vi "LS Acquisition Main (RT).vi"() -> ()   [LabVIEW 2013]
uses:
  Type Defs/Controller List.ctl
  Type Defs/Controller Names.ctl
  Controls/Alarm Config.ctl
  Controls/Alarm Definition.ctl
  Controls/Alarm Profile Config.ctl
  Controls/Tank CMDs.ctl
  Controls/Controller Config.ctl
  Controls/Pump Data.ctl
  Controls/Tank Data.ctl
  Controls/HMI Cluster.ctl
  Controls/HMI Header.ctl
  Controls/HMI Tog Buttons.ctl
  Controls/HMI Mom Buttons.ctl
  Type Defs/LS Data.ctl
  Type Defs/Sequence States.ctl
  Type Defs/LS DAS App Config.ctl
  SubVIs/Data Logger/Data Log Init.ctl
  Controls/App Global Mode.ctl
  <vilib>/FPGAPlugInAG/sbRIO-9626/niLvFpga_Open_sbRIO-9626.vi
  <vilib>/Utility/error.llb/Error Cluster From Error Code.vi
  <vilib>/rvi/errors/niLvFpgaAdjustHostInterfaceError.vi
  <vilib>/rvi/interface/nirviOpenFPGA/nirviOpenFPGA.xnode
  FPGA Bitfiles/LS Acquisition.lvbitx
  <vilib>/rvi/interface/nirviReadWriteControl/nirviReadWriteControl.xnode
  <vilib>/Utility/config.llb/NI_LVConfig.lvlib
  <vilib>/rvi/errors/niLvFpgaMergeErrorWithErrorCode.vi
  NiFpgaLv.dll
panel:
  in  "Data File Name:":string caption="*Data File Name:"
  in  "pb.Run Profile":bool
  in  "Bank 2":T1={"7"=TRUE, "8"=TRUE, "9"=TRUE, "10"=TRUE, "11"=TRUE}
  in  "Bank 1":T2={"1"=TRUE, "2"=TRUE, "3"=TRUE, "4"=TRUE, "5"=TRUE} caption="Present"
  out "Recording":bool
  out "Cycles Completed:":u32=17
  out "Read Inputs (ms)":u32
  out "Update Screen (ms)":u32
  out "Run Step (ms)":u32
  in  "Reset Tab":enum32{"Page 1", "Page 2"}(tab)
  in  "pb.Reset OK":bool
  in  "pb.Reset Cancel":bool
  in  "Save As Tab":enum32{"Page 1", "Page 2"}(tab)
  in  "New Profile Name:":string
  in  "pb.Save As OK":bool
  in  "pb.Save As Cancel":bool
  in  "Alarm Tab":enum32{"Page 1", "Page 2"}(tab)
  in  "Set Time Tab":enum32{"Page 1", "Page 2"}(tab)
  in  "Pump Timers Tab":enum32{"Page 2"}(tab)
  in  "LS Serial Numbers":T3 caption="Serial Numbers"
  out "CPU Usage:":dbl=7.74131899555212 format="%.1f"
  in  "Live Data Tab":enum32{"Page 2", "Page 3"}(tab)=enum."Page 3"
  in  "Reset Anomalies":bool
  in  "Reset Total Cycles":bool
  out "Anomalies (Last Cycle)":i32[](array[numeric]) caption="Anomalies\n(Last Cycle)" format="%#.0f"
  out "Anomalies/Cycle":i32[](array[numeric]) caption="Anomalies/\nCycle" format="%#.0f"
  out "Cycles":u32[](array[numeric]) caption="Powered\nCycles" format="%#.0f"
  out "Anomalies Total":i32[](array[numeric]) caption="Anomalies\nTotal" format="%#.0f"
  out "Steps":u32[](array[numeric]) format="%#.0f"
  out "Total Cycles":u32[](array[numeric]) caption="Total\nPowered\nCycles" format="%#.0f"
  out "Replace SD Card":bool=TRUE
  out "SD Card % Usage":dbl format="%.2g"
  in  "Reset Opens":bool
  out "Opens":i32[](array[numeric]) format="%#.0f"
  in  "Title Tab":enum32{"Page 1", "Page 2"}(tab)
  in  "Title":string="LS Data Acquisition System, v1.9"
  out "Time/Date":string
  in  "Login":bool
  in  "pb.Stop Profile":bool
  in  "Main Tab":enum32{"Main", "Live Graph", "Configure"}(tab)
  in  "Profile based record":bool
  in  "Detection Mode:":u16(ring) items=["Vibration", "Slosh", "Dirt"]
  in  "LS Cycle Time (ms):":dbl=244.0 min=0.1 max=1000.0 step=0.1
  in  "LS On Time (ms):":dbl=4.0 min=0.0 max=1000.0 step=0.01
  in  "Bank 2 Power State:":u16(ring) items=["0 - Off", "1 - On", "2 - Pulsing"]
  in  "Bank 1 Power State:":u16(ring) items=["0 - Off", "1 - On", "2 - Pulsing"]
  in  "CA Number:":string
  in  "Profile Name:":string(combo)="test"
  in  "pb.Save As":bool
  out "Location:":string
  in  "Profile:":string[][](table)=[["1", "216000", "1", "2", "244", "4", "1", "67.6"], ["2", "1800", "0", "0", "244", "4", "1", "10.0"], ["3", "39600", "0", "0", "244", "4", "0", ""], ["4", "1800", "0", "0", "244", "4", "1", ""]]
  out "Recording":bool
  out "Step:":i32=2
  out "Time Left:":dbl=0.21101045608520508
  in  "Bank 2 Record Rate (hz)":enum16{"4.37", "1000"}(ring)
  in  "Graph Selection":T4(ring)
  out "Waveform Chart":dbl(graph)
  in  "Pause":bool
  in  "Bank 2 Voltage Offset:":dbl min=0.0 max=999999.0 step=1.0
  in  "Bank 1 Voltage Offset:":dbl min=0.0 max=999999.0 step=1.0
  in  "Cycle Pts to Avg:":i32=20 min=0 max=999999 step=1
  in  "Cycle Threshold:":dbl=1.6 min=0.0 max=999999.0 step=1.0
  in  "Note Tab":enum32{"Page 1", "Page 2"}(tab)
  in  "Stop Profile Note":string
  in  "pb.Note OK":bool
  in  "pb.Note Cancel":bool
  # "Are you sure you want to reset?"
  # "Enter a new elapsed time."
  # "Level Sensor Monitor"
  # "Level Sensor Monitor"
  # "Have not finished debug:\n     check open log\n     should a profile time stop be added\n     watch CPU, nearing limit"
  # "Record Rate=1kHz"
  # "*"
  # "*"
  # "Data file note as to reason for stopping profile:"
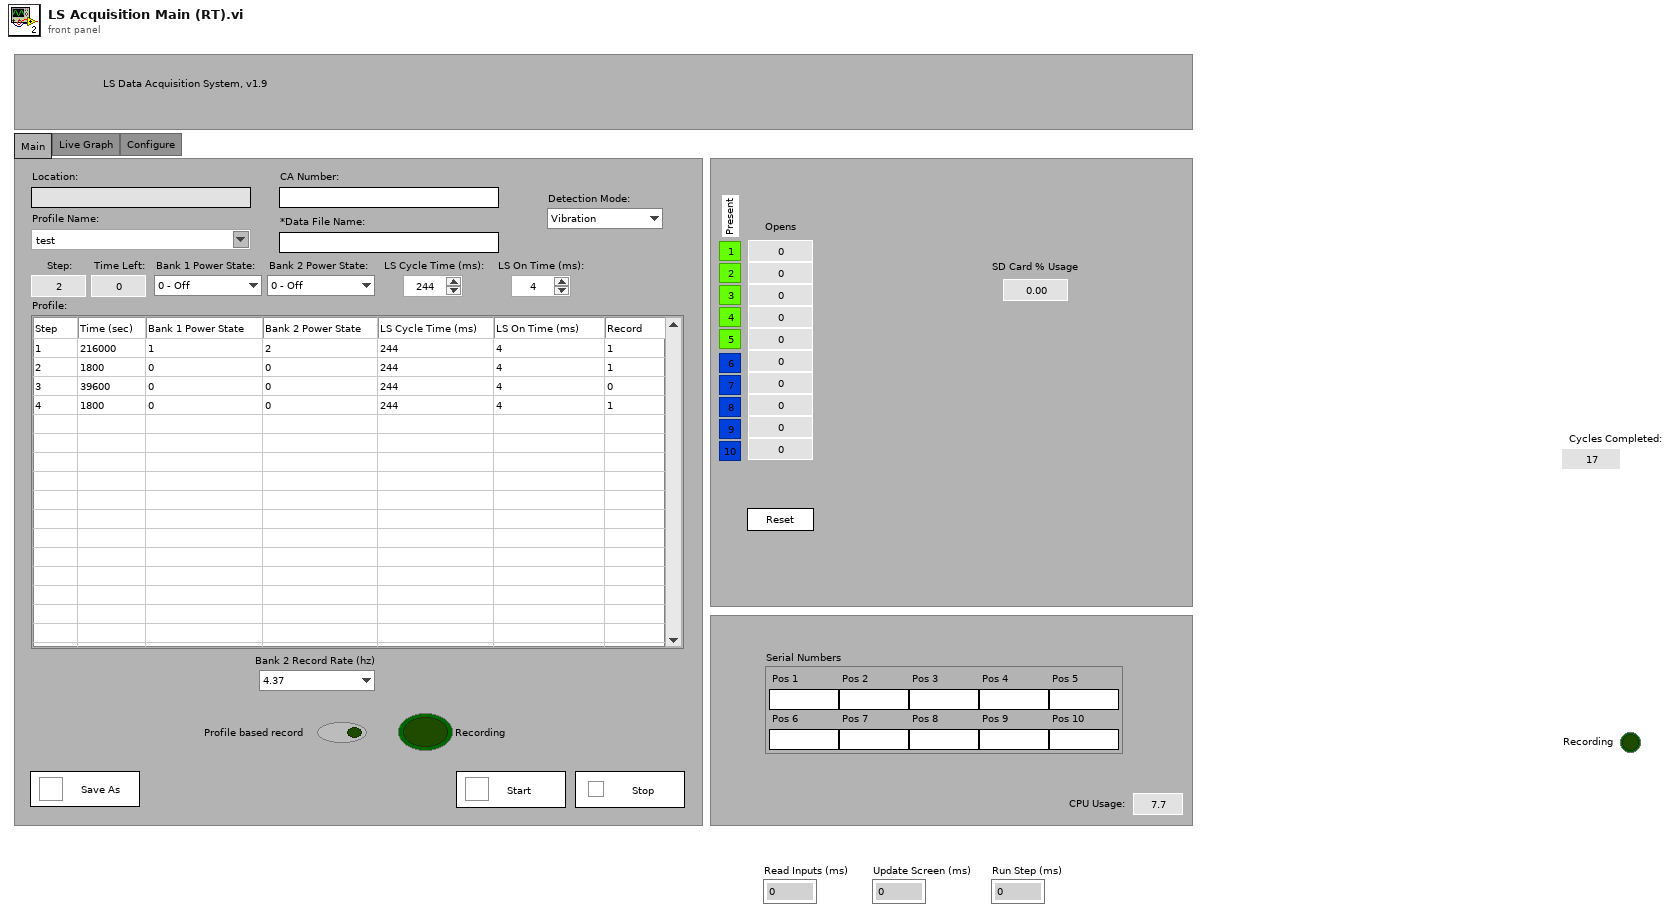
[diagram p1: front panel]
types:
  T1 = cluster{"7":bool, "8":bool, "9":bool, "10":bool, "11":bool}
  T2 = cluster{"1":bool, "2":bool, "3":bool, "4":bool, "5":bool}
  T3 = cluster{"Pos 1":string, "Pos 2":string, "Pos 3":string, "Pos 4":string, "Pos 5":string, "Pos 6":string, "Pos 7":string, "Pos 8":string, "Pos 9":string, "Pos 10":string}
  T4 = enum16{"Pos 1", "Pos 2", "Pos 3", "Pos 4", "Pos 5", "Pos 6", "Pos 7", "Pos 8", "Pos 9", "Pos 10", "Power Supply"}
  T5 = typedef "LS DAS App Config.ctl" = cluster{"Location":string, "Profiles Path":path, "Current Profile":string, "CA Number":string, "Cycles Completed":u32, "Stagger Time (ms)":i32, "Pumps Present":cluster{"Pump 1":bool, "Pump 2":bool, "Pump 3":bool, "Pump 4":bool, "Pump 5":bool, "Pump 6":bool}, "Data Log Init":T6, "Email Handler IP":string, "Cycle Threshold:":dbl, "Cycle Pts to Avg:":i32, "Anomaly Threshold:":dbl, "Normal Steps:":u32, "Step Threshold:":dbl, "Bank 1 Offset":dbl, "Bank 2 Offset":dbl, "LS Power (Freq):":dbl, "LS Power (Duty):":dbl, "Bank 1 Present":cluster{"1":bool, "2":bool, "3":bool, "4":bool, "5":bool}, "Bank 2 Present":cluster{"6":bool, "7":bool, "8":bool, "9":bool, "10":bool}, "Data File Name":string, "Detection Mode":i32, "Serial Numbers":string[], "Profile Record":bool, "Bank2 Record Rate":u16}
  T6 = typedef "Data Log Init.ctl" = cluster{"Data Path":path, "Data Log Rate (S/s)":u32, "AKLH Rate (Hours/S)":dbl, "Sync Time Offset (min)":i32, "IP Last 3":i32, "WebDAV IP":string}
  T7 = typedef "Sequence States.ctl" = enum16{"Main", "Init Files", "Init", "Unused", "Save As", "Start Profile", "Check Step Time", "Alarm", "Alarm Dismiss", "Run Step", "Stop Profile", "Cycle Reset", "Time Reset", "Time Reset All", "Time Set", "Tare CTs", "Save Profile", "Open Profile", "Get Profiles", "Update Screen", "Update Controls", "Save App Config", "Write Outputs", "Disable Background", "Enable Background", "Get/Release Control", "Log Fuel Change", "Fuel Change Popup", "Read Inputs", "Remote Timer Reset", "Controller Change", "Get Alarms", "Init Alarms", "Save Alarms", "Voltage Selection", "Set Watlow Temp 1", "Set Watlow Temp 2", "Get Pressure", "Write Tare Pressure", "Adjust Controls", "Reinit ADC", "Write Initial Times", "Write Pumps Present", "HMI Command", "Save Pump Times", "Check Pump Stop Time", "Save LS App Config", "Init Data File", "Reset LS Cycles", "Reset Anomalies", "Reset Opens", "Save LS Data", "Save LS Test Data", "Check Serial Numbers", "Main Tab", "Allow Data Note", "Resume Profile", "Pause Profile", "Allow Pause Note", "Clear Graph"}
  T8 = typedef "LS Data.ctl" = cluster{"Total Cycles":u32[], "Steps":u32[], "Anomalies Total":i32[], "Cycles":u32[], "Anomalies/Cycle":i32[], "Anomalies (Last Cycle)":i32[], "Opens":i32[]}
  T9 = typedef "HMI Cluster.ctl" = cluster{"Error":errorcluster, "COM Ref":refnum<visa-resource-name>, "Pump Data":T10, "Tank Data":cluster{"PS Actual (V):":dbl, "Temp1":dbl, "Temp2":dbl}, "Power Relays":cluster{"Pump 1":bool, "Pump 2":bool, "Pump 3":bool, "Pump 4":bool, "Pump 5":bool, "Pump 6":bool}, "Pump CMDs":dbl[], "HMI Header":T11, "Tank CMDs":T12, "HMI Tog Buttons":T13, "In Test":bool, "HMI Command":bool, "HMI Mom Buttons":T14, "Controller Config":T15, "Alarm":bool, "Alarm Message 1":string, "Alarm Message 2":string, "Recording":bool, "Serial Numbers":string[], "Pumps Present":bool[]}
  T10 = typedef "Pump Data.ctl" = cluster{"Voltages":dbl[], "PumpCurrent":dbl[], "Speed":dbl[], "ControllerCurrent":dbl[], "Pressure":dbl[], "Flow":dbl[], "Elapsed Time (Display)":dbl[], "Avg Pressure":dbl, "Avg Speed":dbl, "Elapsed Time":dbl[]}
  T11 = typedef "HMI Header.ctl" = cluster{"Line 1":string, "Line 2":string, "Line 3":string, "Line 4":string}
  T12 = typedef "Tank CMDs.ctl" = cluster{"PS CMD":dbl, "Press CMD":dbl, "Temp 1 CMD":dbl, "Temp 2 CMD":dbl}
  T13 = typedef "HMI Tog Buttons.ctl" = cluster{"Start Test":bool, "Toggle Spare 1":bool, "Toggle Spare 2":bool, "Toggle Spare 3":bool, "Toggle Spare 4":bool, "Toggle Spare 5":bool}
  T14 = typedef "HMI Mom Buttons.ctl" = cluster{"Stop":bool, "Reset Timers":bool, "Log Fuel Change":bool, "Alarm Dismiss":bool}
  T15 = typedef "Controller Config.ctl" = cluster{"Controller Name":T16, "CommSeg":i32, "PWM?":bool, "Frequency":i32, "Low Command":dbl, "High Command":dbl, "Stop Command":dbl, "Command Step":dbl, "Solenoid Stop?":bool, "Controller?":bool, "Invert PWM":bool}
  T16 = typedef "Controller Names.ctl" = enum16{"Kuhnke", "Helbako BLDC", "Conti", "Hella BLDC OL PWM", "Hella BLDC Turbine OL PWM", "Hella BLDC Pressure", "Helbako (old)", "TI PWM", "PSA", "Hella Gas", "Hella Diesel", "8 Comm", "10 Comm", "8 Comm Hella", "10 Comm Hella", "8 Comm Omron", "10 Comm Omron", "8 Comm Nissan", "10 Comm Nissan"}
  T17 = typedef "Tank Data.ctl" = cluster{"PS Actual (V):":dbl, "Temp1":dbl, "Temp2":dbl}
  T18 = typedef "Alarm Config.ctl" = cluster{"Alarms:":T19[], "Profile Sync:":T20}
  T19 = typedef "Alarm Definition.ctl" = cluster{"Description:":string, "Enabled:":bool, "Data Index:":i32, "Data Type:":string, "Low Limit:":dbl, "High Limit:":dbl, "Trip Time:":u32, "Profile Sync:":bool}
  T20 = typedef "Alarm Profile Config.ctl" = cluster{"Trip Time:":u32, "Consecutive Trips:":i32}
  T21 = typedef "Controller List.ctl" = cluster{"Controller Name":T16, "CommSeg":i32, "PWM?":bool, "Frequency":i32, "Low Command":dbl, "High Command":dbl, "Stop Command":dbl, "Command Step":dbl, "Solenoid Stop?":bool, "Controller?":bool, "Invert PWM":bool}[]
  T22 = cluster{"Pump 1":bool, "Pump 2":bool, "Pump 3":bool, "Pump 4":bool, "Pump 5":bool, "Pump 6":bool}
  T23 = cluster{"Error":errorcluster, "Profile":string[][], "LS DAS Config":T5, "Profiles":string[], "Current Step":i32, "Step Time Left":dbl, "Run Profile":bool, "Step Start Time":dbl, "Step Time":dbl, " # of Steps":i32, "Screen Timer":u32, "Last Profile Time":dbl, "Controller CMDs":dbl[], "Client?":bool, "pb.Run Profile":bool, "pb.Resets":bool[], "pb.Sets":bool[], "Initial Times":dbl[], "Pressure Offsets":dbl[], "Login":bool, "Stagger Counter":i32, "New Step":bool, "Inputs Timer":u32, "Tank Data":T17, "Voltage Enable":bool, "Power Relay":cluster{"Pump 1":bool, "Pump 2":bool, "Pump 3":bool, "Pump 4":bool, "Pump 5":bool, "Pump 6":bool}, "Ignition Relay":cluster{"Pump 1":bool, "Pump 2":bool, "Pump 3":bool, "Pump 4":bool, "Pump 5":bool, "Pump 6":bool}, "Controller List":T21, "Alarm Config":T18, "Alarm Config Path":path, "Trip Counters":i32[], "Previous Times":u32[], "Alarm Message 1":string, "Alarm Message 2":string, "Prev ON Times":u32[], "CalArray":dbl[][], "Tank CMDs":T12, "Controller Config":T15, "Fuel Log Path":path, "Pump Data":T10, "Alarm Latch":bool, "Time/Date":string, "Recording":bool, "HMI":T9, "WebDAV Push":bool, "Email Alarms Disabled":bool, "Concat Data":bool, "LS Data":T8, "Main Tab":enum32{"Main", "Live Graph", "Configure"}, "Bank 1 State:":u16, "Bank 2 State:":u16, "LS Data Filepath":path, "Initial LS Data":T8, "day of month":i32, "Pause Test":bool, "ProfileMinute":i32, "Record Step":bool, "Graph Selection":enum16{"Pos 1", "Pos 2", "Pos 3", "Pos 4", "Pos 5", "Pos 6", "Pos 7", "Pos 8", "Pos 9", "Pos 10", "Power Supply"}, "Graph Pause":bool}
  T24 = typedef "App Global Mode.ctl" = enum16{"Read", "Write Client", "Write Login"}
  T25 = enum16{"Read", "Engine Writes", "Main Writes", "Write Anomalies", "Write Init Data", "Write Storage", "Write Note", "Read Note"}
  T26 = cluster{"Running?":bool, "Record":bool, "Data Filepath":path, "Serial Numbers":string[]}
  T27 = enum32{"Main", "Live Graph", "Configure", "Alarms", "Advanced"}
  T28 = enum8{"Enabled", "Disabled", "Disabled and Grayed Out"}
  T29 = cluster{"6":bool, "7":bool, "8":bool, "9":bool, "10":bool}
  T30 = typedef "NI_LVConfig.lvlib/Config Data RefNum.ctl" = refnum<k1>
  T31 = typedef "LVDateTimeRec.ctl" = cluster{"fractional second":dbl, "second":i32, "minute":i32, "hour":i32, "day of month":i32, "month":i32, "year":i32, "day of week":i32, "day of year":i32, "DST":i32}
  T32 = cluster{"Serial Numbers[0]":string, "Serial Numbers[1]":string, "Serial Numbers[2]":string, "Serial Numbers[3]":string, "Serial Numbers[4]":string, "Serial Numbers[5]":string, "Serial Numbers[6]":string, "Serial Numbers[7]":string, "Serial Numbers[8]":string, "Serial Numbers[9]":string}
  T33 = cluster{"[0]":string, "[1]":string, "[2]":string, "[3]":string, "[4]":string, "[5]":string, "[6]":string, "[7]":string, "[8]":string, "[9]":string}
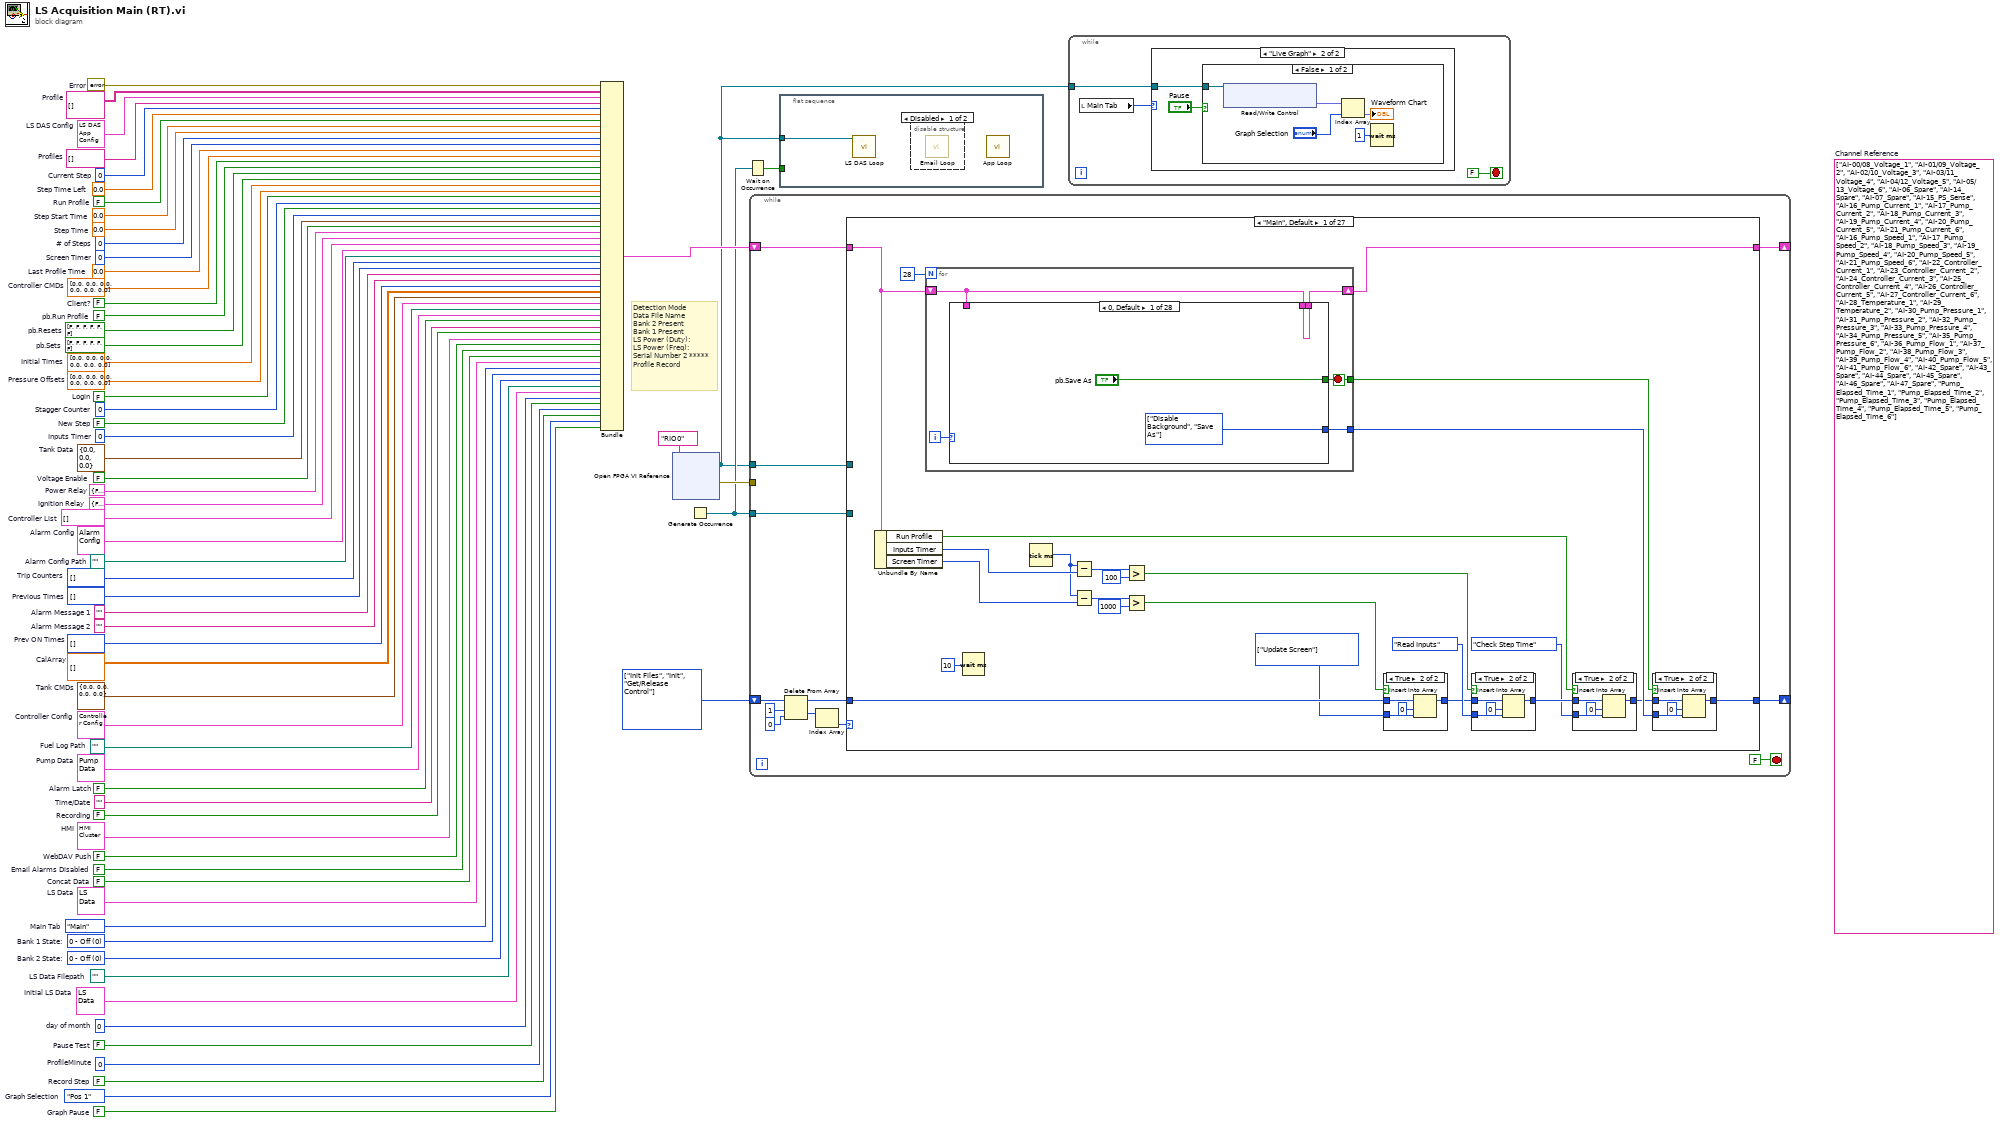
[diagram p0: block diagram]
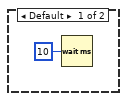
[diagram p2: hidden frame]
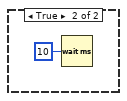
[diagram p3: hidden frame]
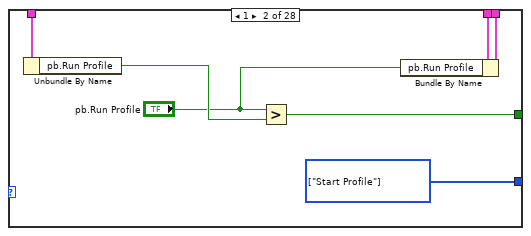
[diagram p9: hidden frame]
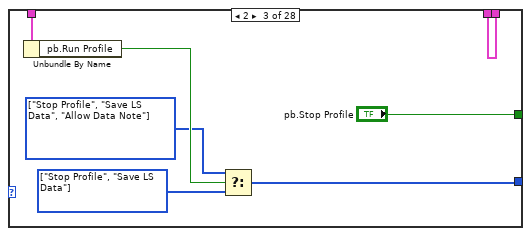
[diagram p10: hidden frame]
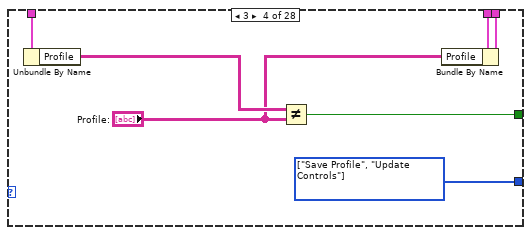
[diagram p11: hidden frame]
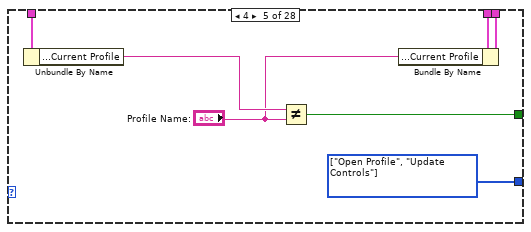
[diagram p12: hidden frame]
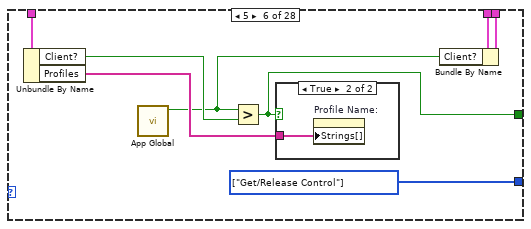
[diagram p13: hidden frame]
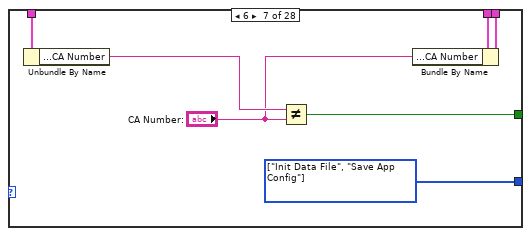
[diagram p15: hidden frame]
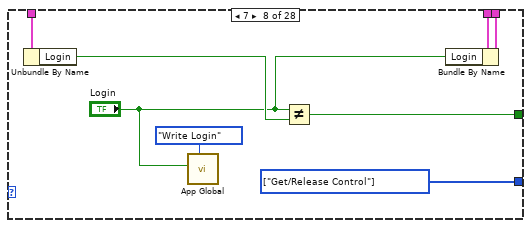
[diagram p16: hidden frame]
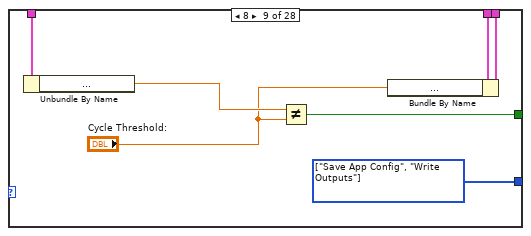
[diagram p17: hidden frame]
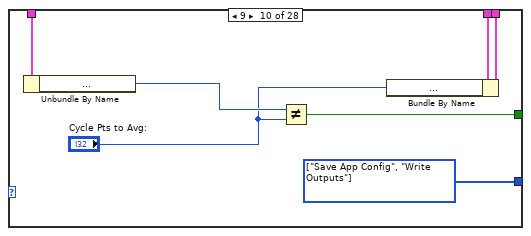
[diagram p18: hidden frame]
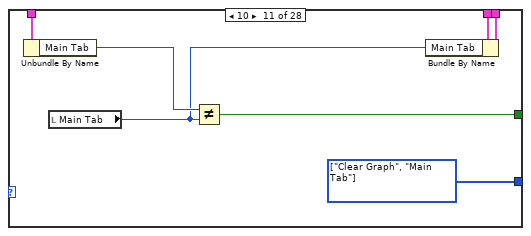
[diagram p19: hidden frame]
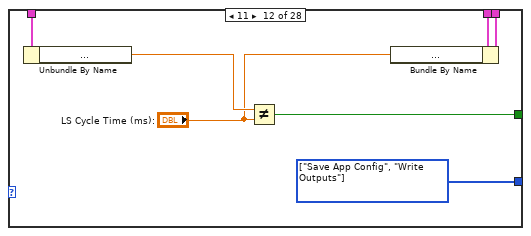
[diagram p20: hidden frame]
diagram:
  w1 = FALSE  # Graph Pause
  w2 = T4."Pos 1"  # Graph Selection
  w3 = enum32{"Main", "Live Graph", "Configure"}."Main"  # Main Tab
  w4 = FALSE  # Record Step
  w5 = T5 {"Location"="", "Profiles Path"=path "", "Current Profile"="", "CA Number"="", "Cycles Completed"=0, "Stagger Time (ms)"=0, "Pumps Present"={"Pump 1"=FALSE, "Pump 2"=FALSE, "Pump 3"=FALSE, "Pump 4"=FALSE, "Pump 5"=FALSE, "Pump 6"=FALSE}, "Data Log Init"={"Data Path"=path "", "Data Log Rate (S/s)"=0, "AKLH Rate (Hours/S)"=0.0, "Sync Time Offset (min)"=0, "IP Last 3"=0, "WebDAV IP"=""}, "Email Handler IP"="", "Cycle Threshold:"=0.0, "Cycle Pts to Avg:"=0, "Anomaly Threshold:"=0.0, "Normal Steps:"=0, "Step Threshold:"=0.0, "Bank 1 Offset"=0.0, "Bank 2 Offset"=0.0, "LS Power (Freq):"=0.0, "LS Power (Duty):"=0.0, "Bank 1 Present"={"1"=FALSE, "2"=FALSE, "3"=FALSE, "4"=FALSE, "5"=FALSE}, "Bank 2 Present"={"6"=FALSE, "7"=FALSE, "8"=FALSE, "9"=FALSE, "10"=FALSE}, "Data File Name"="", "Detection Mode"=0, "Serial Numbers"=[], "Profile Record"=FALSE, "Bank2 Record Rate"=0}  # LS DAS Config
  w6 = 0  # ProfileMinute
  w7 = FALSE  # Pause Test
  w8 = 0  # day of month
  (unwired) string[] ["AI-00/08_Voltage_1", "AI-01/09_Voltage_2", "AI-02/10_Voltage_3", "AI-03/11_Voltage_4", "AI-04/12_Voltage_5", "AI-05/13_Voltage_6", "AI-06_Spare", "AI-14_Spare", "AI-07_Spare", "AI-15_PS_Sense", "AI-16_Pump_Current_1", "AI-17_Pump_Current_2", "AI-18_Pump_Current_3", "AI-19_Pump_Current_4", "AI-20_Pump_Current_5", "AI-21_Pump_Current_6", "AI-16_Pump_Speed_1", "AI-17_Pump_Speed_2", "AI-18_Pump_Speed_3", "AI-19_Pump_Speed_4", "AI-20_Pump_Speed_5", "AI-21_Pump_Speed_6", "AI-22_Controller_Current_1", "AI-23_Controller_Current_2", "AI-24_Controller_Current_3", "AI-25_Controller_Current_4", "AI-26_Controller_Current_5", "AI-27_Controller_Current_6", "AI-28_Temperature_1", "AI-29_Temperature_2", "AI-30_Pump_Pressure_1", "AI-31_Pump_Pressure_2", "AI-32_Pump_Pressure_3", "AI-33_Pump_Pressure_4", "AI-34_Pump_Pressure_5", "AI-35_Pump_Pressure_6", "AI-36_Pump_Flow_1", "AI-37_Pump_Flow_2", "AI-38_Pump_Flow_3", "AI-39_Pump_Flow_4", "AI-40_Pump_Flow_5", "AI-41_Pump_Flow_6", "AI-42_Spare", "AI-43_Spare", "AI-44_Spare", "AI-45_Spare", "AI-46_Spare", "AI-47_Spare", "Pump_Elapsed_Time_1", "Pump_Elapsed_Time_2", "Pump_Elapsed_Time_3", "Pump_Elapsed_Time_4", "Pump_Elapsed_Time_5", "Pump_Elapsed_Time_6"]  # Channel Reference
  w14 = T7[] [enum."Init Files", enum."Init", enum."Get/Release Control"] items=["Main", "Init Files", "Init", "Unused", "Save As", "Start Profile", "Check Step Time", "Alarm", "Alarm Dismiss", "Run Step", "Stop Profile", "Cycle Reset", "Time Reset", "Time Reset All", "Time Set", "Tare CTs", "Save Profile", "Open Profile", "Get Profiles", "Update Screen", "Update Controls", "Save App Config", "Write Outputs", "Disable Background", "Enable Background", "Get/Release Control", "Log Fuel Change", "Fuel Change Popup", "Read Inputs", "Remote Timer Reset", "Controller Change", "Get Alarms", "Init Alarms", "Save Alarms", "Voltage Selection", "Set Watlow Temp 1", "Set Watlow Temp 2", "Get Pressure", "Write Tare Pressure", "Adjust Controls", "Reinit ADC", "Write Initial Times", "Write Pumps Present", "HMI Command", "Save Pump Times", "Check Pump Stop Time", "Save LS App Config", "Init Data File", "Reset LS Cycles", "Reset Anomalies", "Reset Opens", "Save LS Data", "Save LS Test Data", "Check Serial Numbers", "Main Tab", "Allow Data Note", "Resume Profile", "Pause Profile", "Allow Pause Note", "Clear Graph"]
  w15 = T8 {"Total Cycles"=[0, 0, 0, 0, 0, 0, 0, 0, 0, 0, 0, 0], "Steps"=[0, 0, 0, 0, 0, 0, 0, 0, 0, 0, 0, 0], "Anomalies Total"=[0, 0, 0, 0, 0, 0, 0, 0, 0, 0, 0, 0], "Cycles"=[0, 0, 0, 0, 0, 0, 0, 0, 0, 0, 0, 0], "Anomalies/Cycle"=[0, 0, 0, 0, 0, 0, 0, 0, 0, 0, 0, 0], "Anomalies (Last Cycle)"=[0, 0, 0, 0, 0, 0, 0, 0, 0, 0, 0, 0], "Opens"=[0, 0, 0, 0, 0, 0, 0, 0, 0, 0, 0, 0]}  # Initial LS Data
  w16 = path ""  # LS Data Filepath
  w18 = u16 0 items=["0 - Off", "1 - On", "2 - Pulsing"]  # Bank 1 State:
  w17 = u16 0 items=["0 - Off", "1 - On", "2 - Pulsing"]  # Bank 2 State:
  w19 = T8 {"Total Cycles"=[0, 0, 0, 0, 0, 0, 0, 0, 0, 0, 0, 0], "Steps"=[0, 0, 0, 0, 0, 0, 0, 0, 0, 0, 0, 0], "Anomalies Total"=[0, 0, 0, 0, 0, 0, 0, 0, 0, 0, 0, 0], "Cycles"=[0, 0, 0, 0, 0, 0, 0, 0, 0, 0, 0, 0], "Anomalies/Cycle"=[0, 0, 0, 0, 0, 0, 0, 0, 0, 0, 0, 0], "Anomalies (Last Cycle)"=[0, 0, 0, 0, 0, 0, 0, 0, 0, 0, 0, 0], "Opens"=[]}  # LS Data
  w20 = FALSE  # Concat Data
  w21 = FALSE  # Email Alarms Disabled
  w22 = FALSE  # WebDAV Push
  w23 = T9 {"Error"={"status"=FALSE, "code"=0, "source"=""}, "COM Ref"="", "Pump Data"={"Voltages"=[], "PumpCurrent"=[], "Speed"=[], "ControllerCurrent"=[], "Pressure"=[], "Flow"=[], "Elapsed Time (Display)"=[], "Avg Pressure"=0.0, "Avg Speed"=0.0, "Elapsed Time"=[]}, "Tank Data"={"PS Actual (V):"=0.0, "Temp1"=0.0, "Temp2"=0.0}, "Power Relays"={"Pump 1"=FALSE, "Pump 2"=FALSE, "Pump 3"=FALSE, "Pump 4"=FALSE, "Pump 5"=FALSE, "Pump 6"=FALSE}, "Pump CMDs"=[], "HMI Header"={"Line 1"="", "Line 2"="", "Line 3"="", "Line 4"=""}, "Tank CMDs"={"PS CMD"=0.0, "Press CMD"=0.0, "Temp 1 CMD"=0.0, "Temp 2 CMD"=0.0}, "HMI Tog Buttons"={"Start Test"=FALSE, "Toggle Spare 1"=FALSE, "Toggle Spare 2"=FALSE, "Toggle Spare 3"=FALSE, "Toggle Spare 4"=FALSE, "Toggle Spare 5"=FALSE}, "In Test"=FALSE, "HMI Command"=FALSE, "HMI Mom Buttons"={"Stop"=FALSE, "Reset Timers"=FALSE, "Log Fuel Change"=FALSE, "Alarm Dismiss"=FALSE}, "Controller Config"={"Controller Name"=enum."Kuhnke", "CommSeg"=0, "PWM?"=FALSE, "Frequency"=0, "Low Command"=0.0, "High Command"=0.0, "Stop Command"=0.0, "Command Step"=0.0, "Solenoid Stop?"=FALSE, "Controller?"=FALSE, "Invert PWM"=FALSE}, "Alarm"=FALSE, "Alarm Message 1"="", "Alarm Message 2"="", "Recording"=FALSE, "Serial Numbers"=[], "Pumps Present"=[]}  # HMI
  w24 = T17 {"PS Actual (V):"=0.0, "Temp1"=0.0, "Temp2"=0.0}  # Tank Data
  w25 = FALSE  # Recording
  w26 = ""  # Time/Date
  w27 = ""  # Alarm Message 2
  w28 = FALSE  # Alarm Latch
  w29 = T10 {"Voltages"=[0.015201568603515625, 0.00335693359375, 0.003021240234375, 0.12260055541992188, 0.06085968017578125, 0.052234649658203125], "PumpCurrent"=[0.015201568603515625, 0.00335693359375, 0.003021240234375, 0.12260055541992188, 0.06085968017578125, 0.052234649658203125], "Speed"=[0.0, 0.0, 0.0, 0.0, 0.0, 0.0], "ControllerCurrent"=[0.015201568603515625, 0.00335693359375, 0.003021240234375, 0.12260055541992188, 0.06085968017578125, 0.052234649658203125], "Pressure"=[0.015201568603515625, 0.00335693359375, 0.003021240234375, 0.12260055541992188, 0.06085968017578125, 0.052234649658203125], "Flow"=[0.0, 0.0, 0.0, 0.125, 0.0625, 0.0625], "Elapsed Time (Display)"=[7.1, 7.1, 7.1, 458133.45, 458138.85000000003, 458126.75], "Avg Pressure"=0.0, "Avg Speed"=0.0, "Elapsed Time"=[]}  # Pump Data
  w30 = path ""  # Fuel Log Path
  w31 = T15 {"Controller Name"=enum."Kuhnke", "CommSeg"=0, "PWM?"=FALSE, "Frequency"=0, "Low Command"=0.0, "High Command"=0.0, "Stop Command"=0.0, "Command Step"=0.0, "Solenoid Stop?"=FALSE, "Controller?"=FALSE, "Invert PWM"=FALSE}  # Controller Config
  w32 = T12 {"PS CMD"=0.0, "Press CMD"=0.0, "Temp 1 CMD"=0.0, "Temp 2 CMD"=0.0}  # Tank CMDs
  w33 = dbl[][] []  # CalArray
  w34 = u32[] []  # Prev ON Times
  w35 = ""  # Alarm Message 1
  w36 = u32[] []  # Previous Times
  w37 = i32[] []  # Trip Counters
  w38 = path ""  # Alarm Config Path
  w39 = T18 {"Alarms:"=[{"Description:"="", "Enabled:"=FALSE, "Data Index:"=0, "Data Type:"="", "Low Limit:"=0.0, "High Limit:"=0.0, "Trip Time:"=0, "Profile Sync:"=FALSE}, {"Description:"="", "Enabled:"=FALSE, "Data Index:"=0, "Data Type:"="", "Low Limit:"=0.0, "High Limit:"=0.0, "Trip Time:"=0, "Profile Sync:"=FALSE}, {"Description:"="", "Enabled:"=FALSE, "Data Index:"=0, "Data Type:"="", "Low Limit:"=0.0, "High Limit:"=0.0, "Trip Time:"=0, "Profile Sync:"=FALSE}, {"Description:"="", "Enabled:"=FALSE, "Data Index:"=0, "Data Type:"="", "Low Limit:"=0.0, "High Limit:"=0.0, "Trip Time:"=0, "Profile Sync:"=FALSE}, {"Description:"="", "Enabled:"=FALSE, "Data Index:"=0, "Data Type:"="", "Low Limit:"=0.0, "High Limit:"=0.0, "Trip Time:"=0, "Profile Sync:"=FALSE}, {"Description:"="", "Enabled:"=FALSE, "Data Index:"=0, "Data Type:"="", "Low Limit:"=0.0, "High Limit:"=0.0, "Trip Time:"=0, "Profile Sync:"=FALSE}, {"Description:"="", "Enabled:"=FALSE, "Data Index:"=0, "Data Type:"="", "Low Limit:"=0.0, "High Limit:"=0.0, "Trip Time:"=0, "Profile Sync:"=FALSE}, {"Description:"="", "Enabled:"=FALSE, "Data Index:"=0, "Data Type:"="", "Low Limit:"=0.0, "High Limit:"=0.0, "Trip Time:"=0, "Profile Sync:"=FALSE}], "Profile Sync:"={"Trip Time:"=0, "Consecutive Trips:"=0}}  # Alarm Config
  w40 = T21 []  # Controller List
  w41 = T22 {"Pump 1"=FALSE, "Pump 2"=FALSE, "Pump 3"=FALSE, "Pump 4"=FALSE, "Pump 5"=FALSE, "Pump 6"=FALSE}  # Ignition Relay
  w42 = T22 {"Pump 1"=FALSE, "Pump 2"=FALSE, "Pump 3"=FALSE, "Pump 4"=FALSE, "Pump 5"=FALSE, "Pump 6"=FALSE}  # Power Relay
  w43 = FALSE  # Voltage Enable
  w44 = u32 0  # Inputs Timer
  w45 = dbl[] [0.0, 0.0, 0.0, 0.0, 0.0, 0.0]  # Pressure Offsets
  w47 = FALSE  # New Step
  w48 = 0  # Stagger Counter
  w49 = FALSE  # Login
  w50 = dbl[] [0.0, 0.0, 0.0, 0.0, 0.0, 0.0]  # Initial Times
  w51 = bool[] [FALSE, FALSE, FALSE, FALSE, FALSE, FALSE]  # pb.Sets
  w52 = bool[] [FALSE, FALSE, FALSE, FALSE, FALSE, FALSE]  # pb.Resets
  w53 = FALSE  # pb.Run Profile
  w54 = FALSE  # Client?
  w55 = dbl[] [0.0, 0.0, 0.0, 0.0, 0.0, 0.0]  # Controller CMDs
  w56 = 0.0  # Last Profile Time
  w57 = u32 0  # Screen Timer
  w58 = 0  # # of Steps
  w59 = 0.0  # Step Time
  w60 = 0.0  # Step Start Time
  w61 = FALSE  # Run Profile
  w63 = 0  # Current Step
  w62 = 0.0  # Step Time Left
  w64 = string[] []  # Profiles
  w65 = string[][] []  # Profile
  w66 = errorcluster {"status"=FALSE, "code"=0, "source"=""}  # Error
  # "Detection Mode\nData File Name\nBank 2 Present\nBank 1 Present\nLS Power (Duty):\nLS Power (Freq):\nSerial Number 2 *****\nProfile Record"
  n1 = Bundle("Error"=w66, "Profile"=w65, "LS DAS Config"=w5, "Profiles"=w64, "Current Step"=w63, "Step Time Left"=w62, "Run Profile"=w61, "Step Start Time"=w60, "Step Time"=w59, "# of Steps"=w58, "Screen Timer"=w57, "Last Profile Time"=w56, "Controller CMDs"=w55, "Client?"=w54, "pb.Run Profile"=w53, "pb.Resets"=w52, "pb.Sets"=w51, "Initial Times"=w50, "Pressure Offsets"=w45, "Login"=w49, "Stagger Counter"=w48, "New Step"=w47, "Inputs Timer"=w44, "Tank Data"=w24, "Voltage Enable"=w43, "Power Relay"=w42, "Ignition Relay"=w41, "Controller List"=w40, "Alarm Config"=w39, "Alarm Config Path"=w38, "Trip Counters"=w37, "Previous Times"=w36, "Alarm Message 1"=w35, "Alarm Message 2"=w27, "Prev ON Times"=w34, "CalArray"=w33, "Tank CMDs"=w32, "Controller Config"=w31, "Fuel Log Path"=w30, "Pump Data"=w29, "Alarm Latch"=w28, "Time/Date"=w26, "Recording"=w25, "HMI"=w23, "WebDAV Push"=w22, "Email Alarms Disabled"=w21, "Concat Data"=w20, "LS Data"=w19, "Main Tab"=w3, "Bank 1 State:"=w18, "Bank 2 State:"=w17, "LS Data Filepath"=w16, "Initial LS Data"=w15, "day of month"=w8, "Pause Test"=w7, "ProfileMinute"=w6, "Record Step"=w4, "Graph Selection"=w2, "Graph Pause"=w1) -> (w46:T23)  [unwired: 1 in]
  n2 = xnode "Open FPGA VI Reference"("resource name"=tag "RIO0") -> ("FPGA VI Reference Out"=w9:refnum<k20>, "error out"=w13:errorcluster)  [unwired: 1 in]
  n3 = Generate Occurrence() -> (w11:refnum<k4>)
  n4 = Wait on Occurrence(2:w11) -> (0:w10:bool)  [unwired: 2 in]
  n5 = while {
    shift-right: [w75] -> _
    shift-left: w14 -> [w73]
    shift-right: [w76] -> _
    shift-left: w46 -> [w77]
    tunnel: w9 -> [w74]
    tunnel: w11 -> [w68]
    tunnel: w13 -> [_]
    stop <- FALSE stop-if-true
    n6 = Delete From Array(array=w73, length=1, index=0 ("length")) -> (deleted portion=w69:T7[], array with subset deleted=w72:T7[])
    n7 = Index Array(array=w69) -> (element=w67:T7)  [unwired: 1 in]
    n8 = case shown="\"Main\", Default" w67 {
      selector: w67 -> [_ _ _ _ _ _ _ _ _ _ _ _ _ _ _ _ _ _ _ w855 _ _ _ _ _ _ _]
      tunnel: [w84 w366 w461 w487 w494 w509 w523 w552 w583 w641 w649 w695 w727 w765 w785 w802 w826 w830 w835 w847 w886 w907 w932 w941 w948 w957 w993] -> w76
      tunnel: w77 -> [w102 w367 w460 w487 w495 w510 w524 w541 w584 w618 w649 w696 w728 w765 w788 w803 w826 w830 w835 w856 w886 w908 w932 w942 w948 w957 w993]
      tunnel: [w97 w329 w452 w486 w488 w499 w519 w545 w553 w616 w648 w693 w709 w752 w791 w797 w827 w829 w833 w853 w885 w909 w931 w940 w949 w960 w992] -> w75
      tunnel: w74 -> [_ _ w417 _ _ _ _ _ _ _ w655 w691 _ _ _ _ _ _ w834 w857 _ _ _ _ _ _ _]
      tunnel: w72 -> [w91 w329 w455 w486 w489 w500 w519 w546 w565 w637 w648 w693 w734 w752 w792 w798 w827 w829 w833 w854 w885 w909 w931 w940 w949 w961 w992]
      tunnel: w68 -> [_ _ w459 _ _ _ _ _ _ _ _ _ _ _ _ _ _ _ _ _ _ _ _ _ _ _ _]
      frame "Main", Default {
        w80 = T7[] [enum."Update Screen"] items=["Main", "Init Files", "Init", "Unused", "Save As", "Start Profile", "Check Step Time", "Alarm", "Alarm Dismiss", "Run Step", "Stop Profile", "Cycle Reset", "Time Reset", "Time Reset All", "Time Set", "Tare CTs", "Save Profile", "Open Profile", "Get Profiles", "Update Screen", "Update Controls", "Save App Config", "Write Outputs", "Disable Background", "Enable Background", "Get/Release Control", "Log Fuel Change", "Fuel Change Popup", "Read Inputs", "Remote Timer Reset", "Controller Change", "Get Alarms", "Init Alarms", "Save Alarms", "Voltage Selection", "Set Watlow Temp 1", "Set Watlow Temp 2", "Get Pressure", "Write Tare Pressure", "Adjust Controls", "Reinit ADC", "Write Initial Times", "Write Pumps Present", "HMI Command", "Save Pump Times", "Check Pump Stop Time", "Save LS App Config", "Init Data File", "Reset LS Cycles", "Reset Anomalies", "Reset Opens", "Save LS Data", "Save LS Test Data", "Check Serial Numbers", "Main Tab", "Allow Data Note", "Resume Profile", "Pause Profile", "Allow Pause Note", "Clear Graph"]
        n9 = Unbundle By Name(w102) -> ("Run Profile"=w83:bool, "Inputs Timer"=w90:u32, "Screen Timer"=w89:u32)
        n10 = for {
          N: 28 -> [_]
          shift-right: [w127] -> w84
          shift-left: w102 -> [w126]
          tunnel: [w125] -> w99
          tunnel: [w124] -> w98
          i -> [w123]
          stop <- w124 stop-if-true
          n11 = case shown="0, Default" w123 {
            tunnel: w126 -> [w128 w137 w144 w151 w158 w166 w174 w181 w188 w195 w202 w209 w216 w225 w234 w241 w248 w257 w264 w271 w274 w277 w280 w286 w295 w302 w310 w328]
            tunnel: [w128 w136 w144 w150 w157 w165 w173 w180 w187 w194 w201 w208 w215 w224 w233 w240 w247 w256 w263 w270 w274 w277 w280 w285 w294 w301 w309 w327] -> w127
            tunnel: w126 -> [_ w135 w142 w149 w156 w164 w172 w178 w186 w193 w203 w210 w217 w226 w235 w242 w249 w258 w265 w272 _ _ _ w287 w293 w300 w308 w326]
            tunnel: [w129 w134 w139 w146 w152 w162 w168 w177 w189 w196 w199 w207 w214 w223 w232 w239 w246 w255 w262 w269 w275 w278 w281 w282 w289 w297 w306 w324] -> w125
            tunnel: ["pb.Save As" w131 "pb.Stop Profile" w147 w154 w160 w170 w179 w185 w192 w198 w204 w212 w218 w228 w237 w244 w250 w259 w267 "Reset Total Cycles" "Reset Anomalies" "Reset Opens" w284 w291 w298 w305 w318] -> w124
            frame 0, Default {
              w129 = T7[] [enum."Disable Background", enum."Save As"] items=["Main", "Init Files", "Init", "Unused", "Save As", "Start Profile", "Check Step Time", "Alarm", "Alarm Dismiss", "Run Step", "Stop Profile", "Cycle Reset", "Time Reset", "Time Reset All", "Time Set", "Tare CTs", "Save Profile", "Open Profile", "Get Profiles", "Update Screen", "Update Controls", "Save App Config", "Write Outputs", "Disable Background", "Enable Background", "Get/Release Control", "Log Fuel Change", "Fuel Change Popup", "Read Inputs", "Remote Timer Reset", "Controller Change", "Get Alarms", "Init Alarms", "Save Alarms", "Voltage Selection", "Set Watlow Temp 1", "Set Watlow Temp 2", "Get Pressure", "Write Tare Pressure", "Adjust Controls", "Reinit ADC", "Write Initial Times", "Write Pumps Present", "HMI Command", "Save Pump Times", "Check Pump Stop Time", "Save LS App Config", "Init Data File", "Reset LS Cycles", "Reset Anomalies", "Reset Opens", "Save LS Data", "Save LS Test Data", "Check Serial Numbers", "Main Tab", "Allow Data Note", "Resume Profile", "Pause Profile", "Allow Pause Note", "Clear Graph"]
            }
            frame 1 {
              w134 = T7[] [enum."Start Profile"] items=["Main", "Init Files", "Init", "Unused", "Save As", "Start Profile", "Check Step Time", "Alarm", "Alarm Dismiss", "Run Step", "Stop Profile", "Cycle Reset", "Time Reset", "Time Reset All", "Time Set", "Tare CTs", "Save Profile", "Open Profile", "Get Profiles", "Update Screen", "Update Controls", "Save App Config", "Write Outputs", "Disable Background", "Enable Background", "Get/Release Control", "Log Fuel Change", "Fuel Change Popup", "Read Inputs", "Remote Timer Reset", "Controller Change", "Get Alarms", "Init Alarms", "Save Alarms", "Voltage Selection", "Set Watlow Temp 1", "Set Watlow Temp 2", "Get Pressure", "Write Tare Pressure", "Adjust Controls", "Reinit ADC", "Write Initial Times", "Write Pumps Present", "HMI Command", "Save Pump Times", "Check Pump Stop Time", "Save LS App Config", "Init Data File", "Reset LS Cycles", "Reset Anomalies", "Reset Opens", "Save LS Data", "Save LS Test Data", "Check Serial Numbers", "Main Tab", "Allow Data Note", "Resume Profile", "Pause Profile", "Allow Pause Note", "Clear Graph"]
              n12 = Unbundle By Name(w135) -> ("pb.Run Profile"=w133:bool)
              n13 = Greater?(x="pb.Run Profile", y=w133) -> (0:w131:bool)
              n14 = Bundle By Name(cluster=w137, "pb.Run Profile"="pb.Run Profile") -> (w136:T23)
            }
            frame 2 {
              w138 = T7[] [enum."Stop Profile", enum."Save LS Data"] items=["Main", "Init Files", "Init", "Unused", "Save As", "Start Profile", "Check Step Time", "Alarm", "Alarm Dismiss", "Run Step", "Stop Profile", "Cycle Reset", "Time Reset", "Time Reset All", "Time Set", "Tare CTs", "Save Profile", "Open Profile", "Get Profiles", "Update Screen", "Update Controls", "Save App Config", "Write Outputs", "Disable Background", "Enable Background", "Get/Release Control", "Log Fuel Change", "Fuel Change Popup", "Read Inputs", "Remote Timer Reset", "Controller Change", "Get Alarms", "Init Alarms", "Save Alarms", "Voltage Selection", "Set Watlow Temp 1", "Set Watlow Temp 2", "Get Pressure", "Write Tare Pressure", "Adjust Controls", "Reinit ADC", "Write Initial Times", "Write Pumps Present", "HMI Command", "Save Pump Times", "Check Pump Stop Time", "Save LS App Config", "Init Data File", "Reset LS Cycles", "Reset Anomalies", "Reset Opens", "Save LS Data", "Save LS Test Data", "Check Serial Numbers", "Main Tab", "Allow Data Note", "Resume Profile", "Pause Profile", "Allow Pause Note", "Clear Graph"]
              w140 = T7[] [enum."Stop Profile", enum."Save LS Data", enum."Allow Data Note"] items=["Main", "Init Files", "Init", "Unused", "Save As", "Start Profile", "Check Step Time", "Alarm", "Alarm Dismiss", "Run Step", "Stop Profile", "Cycle Reset", "Time Reset", "Time Reset All", "Time Set", "Tare CTs", "Save Profile", "Open Profile", "Get Profiles", "Update Screen", "Update Controls", "Save App Config", "Write Outputs", "Disable Background", "Enable Background", "Get/Release Control", "Log Fuel Change", "Fuel Change Popup", "Read Inputs", "Remote Timer Reset", "Controller Change", "Get Alarms", "Init Alarms", "Save Alarms", "Voltage Selection", "Set Watlow Temp 1", "Set Watlow Temp 2", "Get Pressure", "Write Tare Pressure", "Adjust Controls", "Reinit ADC", "Write Initial Times", "Write Pumps Present", "HMI Command", "Save Pump Times", "Check Pump Stop Time", "Save LS App Config", "Init Data File", "Reset LS Cycles", "Reset Anomalies", "Reset Opens", "Save LS Data", "Save LS Test Data", "Check Serial Numbers", "Main Tab", "Allow Data Note", "Resume Profile", "Pause Profile", "Allow Pause Note", "Clear Graph"]
              n15 = Unbundle By Name(w142) -> ("pb.Run Profile"=w141:bool)
              n16 = Select(t=w140, s=w141, f=w138) -> (s? t:f=w139:T7[])
            }
            frame 3 {
              w146 = T7[] [enum."Save Profile", enum."Update Controls"] items=["Main", "Init Files", "Init", "Unused", "Save As", "Start Profile", "Check Step Time", "Alarm", "Alarm Dismiss", "Run Step", "Stop Profile", "Cycle Reset", "Time Reset", "Time Reset All", "Time Set", "Tare CTs", "Save Profile", "Open Profile", "Get Profiles", "Update Screen", "Update Controls", "Save App Config", "Write Outputs", "Disable Background", "Enable Background", "Get/Release Control", "Log Fuel Change", "Fuel Change Popup", "Read Inputs", "Remote Timer Reset", "Controller Change", "Get Alarms", "Init Alarms", "Save Alarms", "Voltage Selection", "Set Watlow Temp 1", "Set Watlow Temp 2", "Get Pressure", "Write Tare Pressure", "Adjust Controls", "Reinit ADC", "Write Initial Times", "Write Pumps Present", "HMI Command", "Save Pump Times", "Check Pump Stop Time", "Save LS App Config", "Init Data File", "Reset LS Cycles", "Reset Anomalies", "Reset Opens", "Save LS Data", "Save LS Test Data", "Check Serial Numbers", "Main Tab", "Allow Data Note", "Resume Profile", "Pause Profile", "Allow Pause Note", "Clear Graph"]
              n17 = Unbundle By Name(w149) -> ("Profile"=w148:string[][])
              n18 = Not Equal?(x=w148, y="Profile:") -> (x != y?=w147:bool)
              n19 = Bundle By Name(cluster=w151, "Profile"="Profile:") -> (w150:T23)
            }
            frame 4 {
              w152 = T7[] [enum."Open Profile", enum."Update Controls"] items=["Main", "Init Files", "Init", "Unused", "Save As", "Start Profile", "Check Step Time", "Alarm", "Alarm Dismiss", "Run Step", "Stop Profile", "Cycle Reset", "Time Reset", "Time Reset All", "Time Set", "Tare CTs", "Save Profile", "Open Profile", "Get Profiles", "Update Screen", "Update Controls", "Save App Config", "Write Outputs", "Disable Background", "Enable Background", "Get/Release Control", "Log Fuel Change", "Fuel Change Popup", "Read Inputs", "Remote Timer Reset", "Controller Change", "Get Alarms", "Init Alarms", "Save Alarms", "Voltage Selection", "Set Watlow Temp 1", "Set Watlow Temp 2", "Get Pressure", "Write Tare Pressure", "Adjust Controls", "Reinit ADC", "Write Initial Times", "Write Pumps Present", "HMI Command", "Save Pump Times", "Check Pump Stop Time", "Save LS App Config", "Init Data File", "Reset LS Cycles", "Reset Anomalies", "Reset Opens", "Save LS Data", "Save LS Test Data", "Check Serial Numbers", "Main Tab", "Allow Data Note", "Resume Profile", "Pause Profile", "Allow Pause Note", "Clear Graph"]
              n20 = Unbundle By Name(w156) -> ("LS DAS Config.Current Profile"=w155:string)
              n21 = Not Equal?(x=w155, y="Profile Name:") -> (x != y?=w154:bool)
              n22 = Bundle By Name(cluster=w158, "LS DAS Config.Current Profile"="Profile Name:") -> (w157:T23)
            }
            frame 5 {
              w162 = T7[] [enum."Get/Release Control"] items=["Main", "Init Files", "Init", "Unused", "Save As", "Start Profile", "Check Step Time", "Alarm", "Alarm Dismiss", "Run Step", "Stop Profile", "Cycle Reset", "Time Reset", "Time Reset All", "Time Set", "Tare CTs", "Save Profile", "Open Profile", "Get Profiles", "Update Screen", "Update Controls", "Save App Config", "Write Outputs", "Disable Background", "Enable Background", "Get/Release Control", "Log Fuel Change", "Fuel Change Popup", "Read Inputs", "Remote Timer Reset", "Controller Change", "Get Alarms", "Init Alarms", "Save Alarms", "Voltage Selection", "Set Watlow Temp 1", "Set Watlow Temp 2", "Get Pressure", "Write Tare Pressure", "Adjust Controls", "Reinit ADC", "Write Initial Times", "Write Pumps Present", "HMI Command", "Save Pump Times", "Check Pump Stop Time", "Save LS App Config", "Init Data File", "Reset LS Cycles", "Reset Anomalies", "Reset Opens", "Save LS Data", "Save LS Test Data", "Check Serial Numbers", "Main Tab", "Allow Data Note", "Resume Profile", "Pause Profile", "Allow Pause Note", "Clear Graph"]
              n23 = Unbundle By Name(w164) -> ("Client?"=w161:bool, "Profiles"=w163:string[])
              n24 = call "App Global.vi"() -> ("Client? OUT"=w159:bool)  [unwired: 9 in, 2 out]
              n25 = Greater?(x=w159, y=w161) -> (0:w160:bool)
              n26 = case shown="True" w160 {
                tunnel: w163 -> [_ w167]
                frame False {
                }
                frame True {
                  n27 = property on="Profile Name:" class="CmbBox"("Strings[]"=w167) -> ()  [unwired: 2 in, 2 out]
                }
              }
              n28 = Bundle By Name(cluster=w166, "Client?"=w159) -> (w165:T23)
            }
            frame 6 {
              w168 = T7[] [enum."Init Data File", enum."Save App Config"] items=["Main", "Init Files", "Init", "Unused", "Save As", "Start Profile", "Check Step Time", "Alarm", "Alarm Dismiss", "Run Step", "Stop Profile", "Cycle Reset", "Time Reset", "Time Reset All", "Time Set", "Tare CTs", "Save Profile", "Open Profile", "Get Profiles", "Update Screen", "Update Controls", "Save App Config", "Write Outputs", "Disable Background", "Enable Background", "Get/Release Control", "Log Fuel Change", "Fuel Change Popup", "Read Inputs", "Remote Timer Reset", "Controller Change", "Get Alarms", "Init Alarms", "Save Alarms", "Voltage Selection", "Set Watlow Temp 1", "Set Watlow Temp 2", "Get Pressure", "Write Tare Pressure", "Adjust Controls", "Reinit ADC", "Write Initial Times", "Write Pumps Present", "HMI Command", "Save Pump Times", "Check Pump Stop Time", "Save LS App Config", "Init Data File", "Reset LS Cycles", "Reset Anomalies", "Reset Opens", "Save LS Data", "Save LS Test Data", "Check Serial Numbers", "Main Tab", "Allow Data Note", "Resume Profile", "Pause Profile", "Allow Pause Note", "Clear Graph"]
              n29 = Unbundle By Name(w172) -> ("LS DAS Config.CA Number"=w171:string)
              n30 = Not Equal?(x=w171, y="CA Number:") -> (x != y?=w170:bool)
              n31 = Bundle By Name(cluster=w174, "LS DAS Config.CA Number"="CA Number:") -> (w173:T23)
            }
            frame 7 {
              w177 = T7[] [enum."Get/Release Control"] items=["Main", "Init Files", "Init", "Unused", "Save As", "Start Profile", "Check Step Time", "Alarm", "Alarm Dismiss", "Run Step", "Stop Profile", "Cycle Reset", "Time Reset", "Time Reset All", "Time Set", "Tare CTs", "Save Profile", "Open Profile", "Get Profiles", "Update Screen", "Update Controls", "Save App Config", "Write Outputs", "Disable Background", "Enable Background", "Get/Release Control", "Log Fuel Change", "Fuel Change Popup", "Read Inputs", "Remote Timer Reset", "Controller Change", "Get Alarms", "Init Alarms", "Save Alarms", "Voltage Selection", "Set Watlow Temp 1", "Set Watlow Temp 2", "Get Pressure", "Write Tare Pressure", "Adjust Controls", "Reinit ADC", "Write Initial Times", "Write Pumps Present", "HMI Command", "Save Pump Times", "Check Pump Stop Time", "Save LS App Config", "Init Data File", "Reset LS Cycles", "Reset Anomalies", "Reset Opens", "Save LS Data", "Save LS Test Data", "Check Serial Numbers", "Main Tab", "Allow Data Note", "Resume Profile", "Pause Profile", "Allow Pause Note", "Clear Graph"]
              n32 = Unbundle By Name(w178) -> ("Login"=w182:bool)
              n33 = call "App Global.vi"("Mode"=App_Global_Mode."Write Login", "Login"="Login") -> ()  [unwired: 7 in, 3 out]
              n34 = Not Equal?(x="Login", y=w182) -> (x != y?=w179:bool)
              n35 = Bundle By Name(cluster=w181, "Login"="Login") -> (w180:T23)
            }
            frame 8 {
              w189 = T7[] [enum."Save App Config", enum."Write Outputs"] items=["Main", "Init Files", "Init", "Unused", "Save As", "Start Profile", "Check Step Time", "Alarm", "Alarm Dismiss", "Run Step", "Stop Profile", "Cycle Reset", "Time Reset", "Time Reset All", "Time Set", "Tare CTs", "Save Profile", "Open Profile", "Get Profiles", "Update Screen", "Update Controls", "Save App Config", "Write Outputs", "Disable Background", "Enable Background", "Get/Release Control", "Log Fuel Change", "Fuel Change Popup", "Read Inputs", "Remote Timer Reset", "Controller Change", "Get Alarms", "Init Alarms", "Save Alarms", "Voltage Selection", "Set Watlow Temp 1", "Set Watlow Temp 2", "Get Pressure", "Write Tare Pressure", "Adjust Controls", "Reinit ADC", "Write Initial Times", "Write Pumps Present", "HMI Command", "Save Pump Times", "Check Pump Stop Time", "Save LS App Config", "Init Data File", "Reset LS Cycles", "Reset Anomalies", "Reset Opens", "Save LS Data", "Save LS Test Data", "Check Serial Numbers", "Main Tab", "Allow Data Note", "Resume Profile", "Pause Profile", "Allow Pause Note", "Clear Graph"]
              n36 = Unbundle By Name(w186) -> ("LS DAS Config.Cycle Threshold:"=w184:dbl)
              n37 = Not Equal?(x=w184, y="Cycle Threshold:") -> (x != y?=w185:bool)
              n38 = Bundle By Name(cluster=w188, "LS DAS Config.Cycle Threshold:"="Cycle Threshold:") -> (w187:T23)
            }
            frame 9 {
              w196 = T7[] [enum."Save App Config", enum."Write Outputs"] items=["Main", "Init Files", "Init", "Unused", "Save As", "Start Profile", "Check Step Time", "Alarm", "Alarm Dismiss", "Run Step", "Stop Profile", "Cycle Reset", "Time Reset", "Time Reset All", "Time Set", "Tare CTs", "Save Profile", "Open Profile", "Get Profiles", "Update Screen", "Update Controls", "Save App Config", "Write Outputs", "Disable Background", "Enable Background", "Get/Release Control", "Log Fuel Change", "Fuel Change Popup", "Read Inputs", "Remote Timer Reset", "Controller Change", "Get Alarms", "Init Alarms", "Save Alarms", "Voltage Selection", "Set Watlow Temp 1", "Set Watlow Temp 2", "Get Pressure", "Write Tare Pressure", "Adjust Controls", "Reinit ADC", "Write Initial Times", "Write Pumps Present", "HMI Command", "Save Pump Times", "Check Pump Stop Time", "Save LS App Config", "Init Data File", "Reset LS Cycles", "Reset Anomalies", "Reset Opens", "Save LS Data", "Save LS Test Data", "Check Serial Numbers", "Main Tab", "Allow Data Note", "Resume Profile", "Pause Profile", "Allow Pause Note", "Clear Graph"]
              n39 = Unbundle By Name(w193) -> ("LS DAS Config.Cycle Pts to Avg:"=w191:i32)
              n40 = Not Equal?(x=w191, y="Cycle Pts to Avg:") -> (x != y?=w192:bool)
              n41 = Bundle By Name(cluster=w195, "LS DAS Config.Cycle Pts to Avg:"="Cycle Pts to Avg:") -> (w194:T23)
            }
            frame 10 {
              w199 = T7[] [enum."Clear Graph", enum."Main Tab"] items=["Main", "Init Files", "Init", "Unused", "Save As", "Start Profile", "Check Step Time", "Alarm", "Alarm Dismiss", "Run Step", "Stop Profile", "Cycle Reset", "Time Reset", "Time Reset All", "Time Set", "Tare CTs", "Save Profile", "Open Profile", "Get Profiles", "Update Screen", "Update Controls", "Save App Config", "Write Outputs", "Disable Background", "Enable Background", "Get/Release Control", "Log Fuel Change", "Fuel Change Popup", "Read Inputs", "Remote Timer Reset", "Controller Change", "Get Alarms", "Init Alarms", "Save Alarms", "Voltage Selection", "Set Watlow Temp 1", "Set Watlow Temp 2", "Get Pressure", "Write Tare Pressure", "Adjust Controls", "Reinit ADC", "Write Initial Times", "Write Pumps Present", "HMI Command", "Save Pump Times", "Check Pump Stop Time", "Save LS App Config", "Init Data File", "Reset LS Cycles", "Reset Anomalies", "Reset Opens", "Save LS Data", "Save LS Test Data", "Check Serial Numbers", "Main Tab", "Allow Data Note", "Resume Profile", "Pause Profile", "Allow Pause Note", "Clear Graph"]
              n42 = Unbundle By Name(w203) -> ("Main Tab"=w200:enum32{"Main", "Live Graph", "Configure"})
              n43 = local read "Main Tab"() -> (w197:enum32{"Main", "Live Graph", "Configure"})
              n44 = Not Equal?(x=w200, y=w197) -> (x != y?=w198:bool)
              n45 = Bundle By Name(cluster=w202, "Main Tab"=w197) -> (w201:T23)
            }
            frame 11 {
              w207 = T7[] [enum."Save App Config", enum."Write Outputs"] items=["Main", "Init Files", "Init", "Unused", "Save As", "Start Profile", "Check Step Time", "Alarm", "Alarm Dismiss", "Run Step", "Stop Profile", "Cycle Reset", "Time Reset", "Time Reset All", "Time Set", "Tare CTs", "Save Profile", "Open Profile", "Get Profiles", "Update Screen", "Update Controls", "Save App Config", "Write Outputs", "Disable Background", "Enable Background", "Get/Release Control", "Log Fuel Change", "Fuel Change Popup", "Read Inputs", "Remote Timer Reset", "Controller Change", "Get Alarms", "Init Alarms", "Save Alarms", "Voltage Selection", "Set Watlow Temp 1", "Set Watlow Temp 2", "Get Pressure", "Write Tare Pressure", "Adjust Controls", "Reinit ADC", "Write Initial Times", "Write Pumps Present", "HMI Command", "Save Pump Times", "Check Pump Stop Time", "Save LS App Config", "Init Data File", "Reset LS Cycles", "Reset Anomalies", "Reset Opens", "Save LS Data", "Save LS Test Data", "Check Serial Numbers", "Main Tab", "Allow Data Note", "Resume Profile", "Pause Profile", "Allow Pause Note", "Clear Graph"]
              n46 = Unbundle By Name(w210) -> ("LS DAS Config.LS Power (Freq):"=w206:dbl)
              n47 = Not Equal?(x=w206, y="LS Cycle Time (ms):") -> (x != y?=w204:bool)
              n48 = Bundle By Name(cluster=w209, "LS DAS Config.LS Power (Freq):"="LS Cycle Time (ms):") -> (w208:T23)
            }
            frame 12 {
              w214 = T7[] [enum."Save App Config", enum."Write Outputs"] items=["Main", "Init Files", "Init", "Unused", "Save As", "Start Profile", "Check Step Time", "Alarm", "Alarm Dismiss", "Run Step", "Stop Profile", "Cycle Reset", "Time Reset", "Time Reset All", "Time Set", "Tare CTs", "Save Profile", "Open Profile", "Get Profiles", "Update Screen", "Update Controls", "Save App Config", "Write Outputs", "Disable Background", "Enable Background", "Get/Release Control", "Log Fuel Change", "Fuel Change Popup", "Read Inputs", "Remote Timer Reset", "Controller Change", "Get Alarms", "Init Alarms", "Save Alarms", "Voltage Selection", "Set Watlow Temp 1", "Set Watlow Temp 2", "Get Pressure", "Write Tare Pressure", "Adjust Controls", "Reinit ADC", "Write Initial Times", "Write Pumps Present", "HMI Command", "Save Pump Times", "Check Pump Stop Time", "Save LS App Config", "Init Data File", "Reset LS Cycles", "Reset Anomalies", "Reset Opens", "Save LS Data", "Save LS Test Data", "Check Serial Numbers", "Main Tab", "Allow Data Note", "Resume Profile", "Pause Profile", "Allow Pause Note", "Clear Graph"]
              n49 = Unbundle By Name(w217) -> ("LS DAS Config.LS Power (Duty):"=w213:dbl)
              n50 = Not Equal?(x=w213, y="LS On Time (ms):") -> (x != y?=w212:bool)
              n51 = Bundle By Name(cluster=w216, "LS DAS Config.LS Power (Duty):"="LS On Time (ms):") -> (w215:T23)
            }
            frame 13 {
              w223 = T7[] [enum."Save App Config", enum."Write Outputs"] items=["Main", "Init Files", "Init", "Unused", "Save As", "Start Profile", "Check Step Time", "Alarm", "Alarm Dismiss", "Run Step", "Stop Profile", "Cycle Reset", "Time Reset", "Time Reset All", "Time Set", "Tare CTs", "Save Profile", "Open Profile", "Get Profiles", "Update Screen", "Update Controls", "Save App Config", "Write Outputs", "Disable Background", "Enable Background", "Get/Release Control", "Log Fuel Change", "Fuel Change Popup", "Read Inputs", "Remote Timer Reset", "Controller Change", "Get Alarms", "Init Alarms", "Save Alarms", "Voltage Selection", "Set Watlow Temp 1", "Set Watlow Temp 2", "Get Pressure", "Write Tare Pressure", "Adjust Controls", "Reinit ADC", "Write Initial Times", "Write Pumps Present", "HMI Command", "Save Pump Times", "Check Pump Stop Time", "Save LS App Config", "Init Data File", "Reset LS Cycles", "Reset Anomalies", "Reset Opens", "Save LS Data", "Save LS Test Data", "Check Serial Numbers", "Main Tab", "Allow Data Note", "Resume Profile", "Pause Profile", "Allow Pause Note", "Clear Graph"]
              n52 = Unbundle By Name(w226) -> ("LS DAS Config.Bank 1 Present"=w222:T2)
              n53 = Not Equal?(x=w222, y="Bank 1") -> (x != y?=w220:T2)
              n54 = Cluster To Array(cluster=w220) -> (array=w219:bool[])
              n55 = Or Array Elements(Boolean array=w219) -> (logical OR=w218:bool)
              n56 = Bundle By Name(cluster=w225, "LS DAS Config.Bank 1 Present"="Bank 1") -> (w224:T23)
            }
            frame 14 {
              w232 = T7[] [enum."Save App Config", enum."Write Outputs"] items=["Main", "Init Files", "Init", "Unused", "Save As", "Start Profile", "Check Step Time", "Alarm", "Alarm Dismiss", "Run Step", "Stop Profile", "Cycle Reset", "Time Reset", "Time Reset All", "Time Set", "Tare CTs", "Save Profile", "Open Profile", "Get Profiles", "Update Screen", "Update Controls", "Save App Config", "Write Outputs", "Disable Background", "Enable Background", "Get/Release Control", "Log Fuel Change", "Fuel Change Popup", "Read Inputs", "Remote Timer Reset", "Controller Change", "Get Alarms", "Init Alarms", "Save Alarms", "Voltage Selection", "Set Watlow Temp 1", "Set Watlow Temp 2", "Get Pressure", "Write Tare Pressure", "Adjust Controls", "Reinit ADC", "Write Initial Times", "Write Pumps Present", "HMI Command", "Save Pump Times", "Check Pump Stop Time", "Save LS App Config", "Init Data File", "Reset LS Cycles", "Reset Anomalies", "Reset Opens", "Save LS Data", "Save LS Test Data", "Check Serial Numbers", "Main Tab", "Allow Data Note", "Resume Profile", "Pause Profile", "Allow Pause Note", "Clear Graph"]
              n57 = Unbundle By Name(w235) -> ("LS DAS Config.Bank 2 Present"=w231:T29)
              n58 = Not Equal?(x=w231, y="Bank 2") -> (x != y?=w230:cluster{bool, bool, bool, bool, bool})
              n59 = Cluster To Array(cluster=w230) -> (array=w229:bool[])
              n60 = Or Array Elements(Boolean array=w229) -> (logical OR=w228:bool)
              n61 = Bundle By Name(cluster=w234, "LS DAS Config.Bank 2 Present"="Bank 2") -> (w233:T23)
            }
            frame 15 {
              w239 = T7[] [enum."Init Data File", enum."Save App Config"] items=["Main", "Init Files", "Init", "Unused", "Save As", "Start Profile", "Check Step Time", "Alarm", "Alarm Dismiss", "Run Step", "Stop Profile", "Cycle Reset", "Time Reset", "Time Reset All", "Time Set", "Tare CTs", "Save Profile", "Open Profile", "Get Profiles", "Update Screen", "Update Controls", "Save App Config", "Write Outputs", "Disable Background", "Enable Background", "Get/Release Control", "Log Fuel Change", "Fuel Change Popup", "Read Inputs", "Remote Timer Reset", "Controller Change", "Get Alarms", "Init Alarms", "Save Alarms", "Voltage Selection", "Set Watlow Temp 1", "Set Watlow Temp 2", "Get Pressure", "Write Tare Pressure", "Adjust Controls", "Reinit ADC", "Write Initial Times", "Write Pumps Present", "HMI Command", "Save Pump Times", "Check Pump Stop Time", "Save LS App Config", "Init Data File", "Reset LS Cycles", "Reset Anomalies", "Reset Opens", "Save LS Data", "Save LS Test Data", "Check Serial Numbers", "Main Tab", "Allow Data Note", "Resume Profile", "Pause Profile", "Allow Pause Note", "Clear Graph"]
              n62 = Unbundle By Name(w242) -> ("LS DAS Config.Data File Name"=w238:string)
              n63 = Not Equal?(x=w238, y="Data File Name:") -> (x != y?=w237:bool)
              n64 = Bundle By Name(cluster=w241, "LS DAS Config.Data File Name"="Data File Name:") -> (w240:T23)
            }
            frame 16 {
              w246 = T7[] [enum."Save App Config"] items=["Main", "Init Files", "Init", "Unused", "Save As", "Start Profile", "Check Step Time", "Alarm", "Alarm Dismiss", "Run Step", "Stop Profile", "Cycle Reset", "Time Reset", "Time Reset All", "Time Set", "Tare CTs", "Save Profile", "Open Profile", "Get Profiles", "Update Screen", "Update Controls", "Save App Config", "Write Outputs", "Disable Background", "Enable Background", "Get/Release Control", "Log Fuel Change", "Fuel Change Popup", "Read Inputs", "Remote Timer Reset", "Controller Change", "Get Alarms", "Init Alarms", "Save Alarms", "Voltage Selection", "Set Watlow Temp 1", "Set Watlow Temp 2", "Get Pressure", "Write Tare Pressure", "Adjust Controls", "Reinit ADC", "Write Initial Times", "Write Pumps Present", "HMI Command", "Save Pump Times", "Check Pump Stop Time", "Save LS App Config", "Init Data File", "Reset LS Cycles", "Reset Anomalies", "Reset Opens", "Save LS Data", "Save LS Test Data", "Check Serial Numbers", "Main Tab", "Allow Data Note", "Resume Profile", "Pause Profile", "Allow Pause Note", "Clear Graph"]
              n65 = Unbundle By Name(w249) -> ("LS DAS Config.Detection Mode"=w245:i32)
              n66 = Not Equal?(x=w245, y="Detection Mode:") -> (x != y?=w244:bool)
              n67 = Bundle By Name(cluster=w248, "LS DAS Config.Detection Mode"="Detection Mode:") -> (w247:T23)
            }
            frame 17 {
              w255 = T7[] [enum."Check Serial Numbers", enum."Save App Config"] items=["Main", "Init Files", "Init", "Unused", "Save As", "Start Profile", "Check Step Time", "Alarm", "Alarm Dismiss", "Run Step", "Stop Profile", "Cycle Reset", "Time Reset", "Time Reset All", "Time Set", "Tare CTs", "Save Profile", "Open Profile", "Get Profiles", "Update Screen", "Update Controls", "Save App Config", "Write Outputs", "Disable Background", "Enable Background", "Get/Release Control", "Log Fuel Change", "Fuel Change Popup", "Read Inputs", "Remote Timer Reset", "Controller Change", "Get Alarms", "Init Alarms", "Save Alarms", "Voltage Selection", "Set Watlow Temp 1", "Set Watlow Temp 2", "Get Pressure", "Write Tare Pressure", "Adjust Controls", "Reinit ADC", "Write Initial Times", "Write Pumps Present", "HMI Command", "Save Pump Times", "Check Pump Stop Time", "Save LS App Config", "Init Data File", "Reset LS Cycles", "Reset Anomalies", "Reset Opens", "Save LS Data", "Save LS Test Data", "Check Serial Numbers", "Main Tab", "Allow Data Note", "Resume Profile", "Pause Profile", "Allow Pause Note", "Clear Graph"]
              n68 = Unbundle By Name(w258) -> ("LS DAS Config.Serial Numbers"=w254:string[])
              n69 = Cluster To Array(cluster="LS Serial Numbers") -> (array=w252:string[])
              n70 = Not Equal?(x=w254, y=w252) -> (x != y?=w251:bool[])
              n71 = Or Array Elements(Boolean array=w251) -> (logical OR=w250:bool)
              n72 = Bundle By Name(cluster=w257, "LS DAS Config.Serial Numbers"=w252) -> (w256:T23)
            }
            frame 18 {
              w262 = T7[] [enum."Write Outputs"] items=["Main", "Init Files", "Init", "Unused", "Save As", "Start Profile", "Check Step Time", "Alarm", "Alarm Dismiss", "Run Step", "Stop Profile", "Cycle Reset", "Time Reset", "Time Reset All", "Time Set", "Tare CTs", "Save Profile", "Open Profile", "Get Profiles", "Update Screen", "Update Controls", "Save App Config", "Write Outputs", "Disable Background", "Enable Background", "Get/Release Control", "Log Fuel Change", "Fuel Change Popup", "Read Inputs", "Remote Timer Reset", "Controller Change", "Get Alarms", "Init Alarms", "Save Alarms", "Voltage Selection", "Set Watlow Temp 1", "Set Watlow Temp 2", "Get Pressure", "Write Tare Pressure", "Adjust Controls", "Reinit ADC", "Write Initial Times", "Write Pumps Present", "HMI Command", "Save Pump Times", "Check Pump Stop Time", "Save LS App Config", "Init Data File", "Reset LS Cycles", "Reset Anomalies", "Reset Opens", "Save LS Data", "Save LS Test Data", "Check Serial Numbers", "Main Tab", "Allow Data Note", "Resume Profile", "Pause Profile", "Allow Pause Note", "Clear Graph"]
              n73 = Unbundle By Name(w265) -> ("Bank 1 State:"=w261:u16)
              n74 = Not Equal?(x=w261, y="Bank 1 Power State:") -> (x != y?=w259:bool)
              n75 = Bundle By Name(cluster=w264, "Bank 1 State:"="Bank 1 Power State:") -> (w263:T23)
            }
            frame 19 {
              w269 = T7[] [enum."Write Outputs"] items=["Main", "Init Files", "Init", "Unused", "Save As", "Start Profile", "Check Step Time", "Alarm", "Alarm Dismiss", "Run Step", "Stop Profile", "Cycle Reset", "Time Reset", "Time Reset All", "Time Set", "Tare CTs", "Save Profile", "Open Profile", "Get Profiles", "Update Screen", "Update Controls", "Save App Config", "Write Outputs", "Disable Background", "Enable Background", "Get/Release Control", "Log Fuel Change", "Fuel Change Popup", "Read Inputs", "Remote Timer Reset", "Controller Change", "Get Alarms", "Init Alarms", "Save Alarms", "Voltage Selection", "Set Watlow Temp 1", "Set Watlow Temp 2", "Get Pressure", "Write Tare Pressure", "Adjust Controls", "Reinit ADC", "Write Initial Times", "Write Pumps Present", "HMI Command", "Save Pump Times", "Check Pump Stop Time", "Save LS App Config", "Init Data File", "Reset LS Cycles", "Reset Anomalies", "Reset Opens", "Save LS Data", "Save LS Test Data", "Check Serial Numbers", "Main Tab", "Allow Data Note", "Resume Profile", "Pause Profile", "Allow Pause Note", "Clear Graph"]
              n76 = Unbundle By Name(w272) -> ("Bank 2 State:"=w268:u16)
              n77 = Not Equal?(x=w268, y="Bank 2 Power State:") -> (x != y?=w267:bool)
              n78 = Bundle By Name(cluster=w271, "Bank 2 State:"="Bank 2 Power State:") -> (w270:T23)
            }
            frame 20 {
              w275 = T7[] [enum."Reset LS Cycles"] items=["Main", "Init Files", "Init", "Unused", "Save As", "Start Profile", "Check Step Time", "Alarm", "Alarm Dismiss", "Run Step", "Stop Profile", "Cycle Reset", "Time Reset", "Time Reset All", "Time Set", "Tare CTs", "Save Profile", "Open Profile", "Get Profiles", "Update Screen", "Update Controls", "Save App Config", "Write Outputs", "Disable Background", "Enable Background", "Get/Release Control", "Log Fuel Change", "Fuel Change Popup", "Read Inputs", "Remote Timer Reset", "Controller Change", "Get Alarms", "Init Alarms", "Save Alarms", "Voltage Selection", "Set Watlow Temp 1", "Set Watlow Temp 2", "Get Pressure", "Write Tare Pressure", "Adjust Controls", "Reinit ADC", "Write Initial Times", "Write Pumps Present", "HMI Command", "Save Pump Times", "Check Pump Stop Time", "Save LS App Config", "Init Data File", "Reset LS Cycles", "Reset Anomalies", "Reset Opens", "Save LS Data", "Save LS Test Data", "Check Serial Numbers", "Main Tab", "Allow Data Note", "Resume Profile", "Pause Profile", "Allow Pause Note", "Clear Graph"]
            }
            frame 21 {
              w278 = T7[] [enum."Reset Anomalies"] items=["Main", "Init Files", "Init", "Unused", "Save As", "Start Profile", "Check Step Time", "Alarm", "Alarm Dismiss", "Run Step", "Stop Profile", "Cycle Reset", "Time Reset", "Time Reset All", "Time Set", "Tare CTs", "Save Profile", "Open Profile", "Get Profiles", "Update Screen", "Update Controls", "Save App Config", "Write Outputs", "Disable Background", "Enable Background", "Get/Release Control", "Log Fuel Change", "Fuel Change Popup", "Read Inputs", "Remote Timer Reset", "Controller Change", "Get Alarms", "Init Alarms", "Save Alarms", "Voltage Selection", "Set Watlow Temp 1", "Set Watlow Temp 2", "Get Pressure", "Write Tare Pressure", "Adjust Controls", "Reinit ADC", "Write Initial Times", "Write Pumps Present", "HMI Command", "Save Pump Times", "Check Pump Stop Time", "Save LS App Config", "Init Data File", "Reset LS Cycles", "Reset Anomalies", "Reset Opens", "Save LS Data", "Save LS Test Data", "Check Serial Numbers", "Main Tab", "Allow Data Note", "Resume Profile", "Pause Profile", "Allow Pause Note", "Clear Graph"]
            }
            frame 22 {
              w281 = T7[] [enum."Reset Opens"] items=["Main", "Init Files", "Init", "Unused", "Save As", "Start Profile", "Check Step Time", "Alarm", "Alarm Dismiss", "Run Step", "Stop Profile", "Cycle Reset", "Time Reset", "Time Reset All", "Time Set", "Tare CTs", "Save Profile", "Open Profile", "Get Profiles", "Update Screen", "Update Controls", "Save App Config", "Write Outputs", "Disable Background", "Enable Background", "Get/Release Control", "Log Fuel Change", "Fuel Change Popup", "Read Inputs", "Remote Timer Reset", "Controller Change", "Get Alarms", "Init Alarms", "Save Alarms", "Voltage Selection", "Set Watlow Temp 1", "Set Watlow Temp 2", "Get Pressure", "Write Tare Pressure", "Adjust Controls", "Reinit ADC", "Write Initial Times", "Write Pumps Present", "HMI Command", "Save Pump Times", "Check Pump Stop Time", "Save LS App Config", "Init Data File", "Reset LS Cycles", "Reset Anomalies", "Reset Opens", "Save LS Data", "Save LS Test Data", "Check Serial Numbers", "Main Tab", "Allow Data Note", "Resume Profile", "Pause Profile", "Allow Pause Note", "Clear Graph"]
            }
            frame 23 {
              w282 = T7[] [enum."Save App Config"] items=["Main", "Init Files", "Init", "Unused", "Save As", "Start Profile", "Check Step Time", "Alarm", "Alarm Dismiss", "Run Step", "Stop Profile", "Cycle Reset", "Time Reset", "Time Reset All", "Time Set", "Tare CTs", "Save Profile", "Open Profile", "Get Profiles", "Update Screen", "Update Controls", "Save App Config", "Write Outputs", "Disable Background", "Enable Background", "Get/Release Control", "Log Fuel Change", "Fuel Change Popup", "Read Inputs", "Remote Timer Reset", "Controller Change", "Get Alarms", "Init Alarms", "Save Alarms", "Voltage Selection", "Set Watlow Temp 1", "Set Watlow Temp 2", "Get Pressure", "Write Tare Pressure", "Adjust Controls", "Reinit ADC", "Write Initial Times", "Write Pumps Present", "HMI Command", "Save Pump Times", "Check Pump Stop Time", "Save LS App Config", "Init Data File", "Reset LS Cycles", "Reset Anomalies", "Reset Opens", "Save LS Data", "Save LS Test Data", "Check Serial Numbers", "Main Tab", "Allow Data Note", "Resume Profile", "Pause Profile", "Allow Pause Note", "Clear Graph"]
              n79 = Unbundle By Name(w287) -> ("LS DAS Config.Profile Record"=w288:bool)
              n80 = Not Equal?(x=w288, y="Profile based record") -> (x != y?=w284:bool)
              n81 = Bundle By Name(cluster=w286, "LS DAS Config.Profile Record"="Profile based record") -> (w285:T23)
            }
            frame 24 {
              w289 = T7[] [enum."Save App Config", enum."Write Outputs"] items=["Main", "Init Files", "Init", "Unused", "Save As", "Start Profile", "Check Step Time", "Alarm", "Alarm Dismiss", "Run Step", "Stop Profile", "Cycle Reset", "Time Reset", "Time Reset All", "Time Set", "Tare CTs", "Save Profile", "Open Profile", "Get Profiles", "Update Screen", "Update Controls", "Save App Config", "Write Outputs", "Disable Background", "Enable Background", "Get/Release Control", "Log Fuel Change", "Fuel Change Popup", "Read Inputs", "Remote Timer Reset", "Controller Change", "Get Alarms", "Init Alarms", "Save Alarms", "Voltage Selection", "Set Watlow Temp 1", "Set Watlow Temp 2", "Get Pressure", "Write Tare Pressure", "Adjust Controls", "Reinit ADC", "Write Initial Times", "Write Pumps Present", "HMI Command", "Save Pump Times", "Check Pump Stop Time", "Save LS App Config", "Init Data File", "Reset LS Cycles", "Reset Anomalies", "Reset Opens", "Save LS Data", "Save LS Test Data", "Check Serial Numbers", "Main Tab", "Allow Data Note", "Resume Profile", "Pause Profile", "Allow Pause Note", "Clear Graph"]
              n82 = Unbundle By Name(w293) -> ("LS DAS Config.Bank 1 Offset"=w292:dbl)
              n83 = Not Equal?(x=w292, y="Bank 1 Voltage Offset:") -> (x != y?=w291:bool)
              n84 = Bundle By Name(cluster=w295, "LS DAS Config.Bank 1 Offset"="Bank 1 Voltage Offset:") -> (w294:T23)
            }
            frame 25 {
              w297 = T7[] [enum."Save App Config", enum."Write Outputs"] items=["Main", "Init Files", "Init", "Unused", "Save As", "Start Profile", "Check Step Time", "Alarm", "Alarm Dismiss", "Run Step", "Stop Profile", "Cycle Reset", "Time Reset", "Time Reset All", "Time Set", "Tare CTs", "Save Profile", "Open Profile", "Get Profiles", "Update Screen", "Update Controls", "Save App Config", "Write Outputs", "Disable Background", "Enable Background", "Get/Release Control", "Log Fuel Change", "Fuel Change Popup", "Read Inputs", "Remote Timer Reset", "Controller Change", "Get Alarms", "Init Alarms", "Save Alarms", "Voltage Selection", "Set Watlow Temp 1", "Set Watlow Temp 2", "Get Pressure", "Write Tare Pressure", "Adjust Controls", "Reinit ADC", "Write Initial Times", "Write Pumps Present", "HMI Command", "Save Pump Times", "Check Pump Stop Time", "Save LS App Config", "Init Data File", "Reset LS Cycles", "Reset Anomalies", "Reset Opens", "Save LS Data", "Save LS Test Data", "Check Serial Numbers", "Main Tab", "Allow Data Note", "Resume Profile", "Pause Profile", "Allow Pause Note", "Clear Graph"]
              n85 = Unbundle By Name(w300) -> ("LS DAS Config.Bank 2 Offset"=w299:dbl)
              n86 = Not Equal?(x=w299, y="Bank 2 Voltage Offset:") -> (x != y?=w298:bool)
              n87 = Bundle By Name(cluster=w302, "LS DAS Config.Bank 2 Offset"="Bank 2 Voltage Offset:") -> (w301:T23)
            }
            frame 26 {
              w306 = T7[] [enum."Save App Config"] items=["Main", "Init Files", "Init", "Unused", "Save As", "Start Profile", "Check Step Time", "Alarm", "Alarm Dismiss", "Run Step", "Stop Profile", "Cycle Reset", "Time Reset", "Time Reset All", "Time Set", "Tare CTs", "Save Profile", "Open Profile", "Get Profiles", "Update Screen", "Update Controls", "Save App Config", "Write Outputs", "Disable Background", "Enable Background", "Get/Release Control", "Log Fuel Change", "Fuel Change Popup", "Read Inputs", "Remote Timer Reset", "Controller Change", "Get Alarms", "Init Alarms", "Save Alarms", "Voltage Selection", "Set Watlow Temp 1", "Set Watlow Temp 2", "Get Pressure", "Write Tare Pressure", "Adjust Controls", "Reinit ADC", "Write Initial Times", "Write Pumps Present", "HMI Command", "Save Pump Times", "Check Pump Stop Time", "Save LS App Config", "Init Data File", "Reset LS Cycles", "Reset Anomalies", "Reset Opens", "Save LS Data", "Save LS Test Data", "Check Serial Numbers", "Main Tab", "Allow Data Note", "Resume Profile", "Pause Profile", "Allow Pause Note", "Clear Graph"]
              n88 = Unbundle By Name(w308) -> ("LS DAS Config.Bank2 Record Rate"=w307:u16, "Initial LS Data"=w303:T8)
              n89 = Not Equal?(x=w307, y="Bank 2 Record Rate (hz)") -> (x != y?=w305:bool)
              n90 = case shown="True" w305 {
                tunnel: "Bank 2 Record Rate (hz)" -> [_ w317]
                tunnel: w303 -> [_ w311]
                frame False {
                }
                frame True {
                  n91 = Equal?(x=enum16{"4.37", "1000"}."4.37" ("Bank 2 Record Rate (hz)"), y=w317) -> (x = y?=w312:bool)
                  n92 = Get Volume Info(11:path "u:/" ("path")) -> (2:w314:i64)  [unwired: 1 in, 5 out]
                  n93 = call "LS DAS Global.vi"("Bank2Slow In"=w312, "Mode"=T25."Write Init Data", "Initial LS Data In"=w311, "SDmax'"=w314) -> ()  [unwired: 5 in, 7 out]
                }
              }
              n94 = Bundle By Name(cluster=w310, "LS DAS Config.Bank2 Record Rate"="Bank 2 Record Rate (hz)") -> (w309:T23)
            }
            frame 27 {
              w324 = T7[] [enum."Clear Graph"] items=["Main", "Init Files", "Init", "Unused", "Save As", "Start Profile", "Check Step Time", "Alarm", "Alarm Dismiss", "Run Step", "Stop Profile", "Cycle Reset", "Time Reset", "Time Reset All", "Time Set", "Tare CTs", "Save Profile", "Open Profile", "Get Profiles", "Update Screen", "Update Controls", "Save App Config", "Write Outputs", "Disable Background", "Enable Background", "Get/Release Control", "Log Fuel Change", "Fuel Change Popup", "Read Inputs", "Remote Timer Reset", "Controller Change", "Get Alarms", "Init Alarms", "Save Alarms", "Voltage Selection", "Set Watlow Temp 1", "Set Watlow Temp 2", "Get Pressure", "Write Tare Pressure", "Adjust Controls", "Reinit ADC", "Write Initial Times", "Write Pumps Present", "HMI Command", "Save Pump Times", "Check Pump Stop Time", "Save LS App Config", "Init Data File", "Reset LS Cycles", "Reset Anomalies", "Reset Opens", "Save LS Data", "Save LS Test Data", "Check Serial Numbers", "Main Tab", "Allow Data Note", "Resume Profile", "Pause Profile", "Allow Pause Note", "Clear Graph"]
              n95 = Unbundle By Name(w326) -> ("Graph Selection"=w325:T4, "Graph Pause"=w322:bool)
              n96 = local read "Graph Selection"() -> (w323:T4)
              n97 = local read "Pause"() -> (w321:bool)
              n98 = Not Equal?(x=w325, y=w323) -> (x != y?=w319:bool)
              n99 = Greater?(x=w322, y=w321) -> (0:w320:bool)
              n100 = Or(x=w319, y=w320) -> (x .or. y?=w318:bool)
              n101 = Bundle By Name(cluster=w328, "Graph Selection"=w323, "Graph Pause"=w321) -> (w327:T23)
            }
          }
        }
        n102 = Wait (ms)(milliseconds to wait=u32 10) -> ()  [unwired: 1 out]
        n103 = Tick Count (ms)() -> (millisecond timer value=w88:u32)
        n104 = Subtract(x=w88, y=w90) -> (x-y=w87:u32)
        n105 = Subtract(x=w88, y=w89) -> (x-y=w86:u32)
        n106 = Greater?(x=w87, y=u32 100) -> (0:w82:bool)
        n107 = Greater?(x=w86, y=u32 1000) -> (0:w81:bool)
        n108 = case shown="True" w81 {
          tunnel: w91 -> [w103 w107]
          tunnel: w80 -> [_ w106]
          tunnel: [w103 w104] -> w92
          frame False {
          }
          frame True {
            n109 = Insert Into Array(array=w107, index=0, new element=w106) -> (w104:T7[])
          }
        }
        n110 = case shown="True" w82 {
          tunnel: w92 -> [w108 w112]
          tunnel: Sequence_States."Read Inputs" -> [_ w111]
          tunnel: [w108 w109] -> w95
          frame False {
          }
          frame True {
            n111 = Insert Into Array(array=w112, index=0, new element=w111) -> (w109:T7[])
          }
        }
        n112 = case shown="True" w83 {
          tunnel: w95 -> [w113 w117]
          tunnel: Sequence_States."Check Step Time" -> [_ w116]
          tunnel: [w113 w114] -> w96
          frame False {
          }
          frame True {
            n113 = Insert Into Array(array=w117, index=0, new element=w116) -> (w114:T7[])
          }
        }
        n114 = case shown="True" w98 {
          tunnel: w96 -> [w118 w122]
          tunnel: w99 -> [_ w121]
          tunnel: [w118 w119] -> w97
          frame False {
          }
          frame True {
            n115 = Insert Into Array(array=w122, index=0, new element=w121) -> (w119:T7[])
          }
        }
      }
      frame "Init Files" {
        w358 = dbl[][] [[0.0, 11.0, 0.0, 0.0, 0.0], [0.0, 11.0, 0.0, 0.0, 0.0], [0.0, 11.0, 0.0, 0.0, 0.0], [0.0, 11.0, 0.0, 0.0, 0.0], [0.0, 11.0, 0.0, 0.0, 0.0], [0.0, 11.0, 0.0, 0.0, 0.0], [0.0, 1.0, 0.0, 0.0, 0.0], [0.0, 1.0, 0.0, 0.0, 0.0], [0.0, 1.0, 0.0, 0.0, 0.0], [0.0, 2.0, 0.0, 0.0, 0.0], [0.0, 1.0, 0.0, 0.0, 0.0], [0.0, 1.0, 0.0, 0.0, 0.0], [0.0, 1.0, 0.0, 0.0, 0.0], [0.0, 1.0, 0.0, 0.0, 0.0], [0.0, 1.0, 0.0, 0.0, 0.0], [0.0, 1.0, 0.0, 0.0, 0.0], [0.0, 1.0, 0.0, 0.0, 0.0], [0.0, 1.0, 0.0, 0.0, 0.0], [0.0, 1.0, 0.0, 0.0, 0.0], [0.0, 1.0, 0.0, 0.0, 0.0], [0.0, 1.0, 0.0, 0.0, 0.0], [0.0, 1.0, 0.0, 0.0, 0.0], [-60.0, 24.0, 0.0, 0.0, 0.0], [-60.0, 24.0, 0.0, 0.0, 0.0], [-60.0, 24.0, 0.0, 0.0, 0.0], [-60.0, 24.0, 0.0, 0.0, 0.0], [-60.0, 24.0, 0.0, 0.0, 0.0], [-60.0, 24.0, 0.0, 0.0, 0.0], [-660.0, 200.0, 0.0, 0.0, 0.0], [-660.0, 200.0, 0.0, 0.0, 0.0], [-258.5, 258.5, 0.0, 0.0, 0.0], [-258.5, 258.5, 0.0, 0.0, 0.0], [-258.5, 258.5, 0.0, 0.0, 0.0], [-258.5, 258.5, 0.0, 0.0, 0.0], [-258.5, 258.5, 0.0, 0.0, 0.0], [-258.5, 258.5, 0.0, 0.0, 0.0], [-150.0, 150.0, 0.0, 0.0, 0.0], [-150.0, 150.0, 0.0, 0.0, 0.0], [-150.0, 150.0, 0.0, 0.0, 0.0], [-150.0, 150.0, 0.0, 0.0, 0.0], [-150.0, 150.0, 0.0, 0.0, 0.0], [-150.0, 150.0, 0.0, 0.0, 0.0], [0.0, 1.0, 0.0, 0.0, 0.0], [0.0, 1.0, 0.0, 0.0, 0.0], [0.0, 1.0, 0.0, 0.0, 0.0], [0.0, 1.0, 0.0, 0.0, 0.0], [0.0, 1.0, 0.0, 0.0, 0.0], [0.0, 1.0, 0.0, 0.0, 0.0], [0.0, 11.0, 0.0, 0.0, 0.0], [0.0, 11.0, 0.0, 0.0, 0.0], [0.0, 11.0, 0.0, 0.0, 0.0], [0.0, 11.0, 0.0, 0.0, 0.0], [0.0, 11.0, 0.0, 0.0, 0.0], [0.0, 11.0, 0.0, 0.0, 0.0], [0.0, 0.0001, 0.0, 0.0, 0.0], [0.0, 0.0001, 0.0, 0.0, 0.0], [0.0, 0.0001, 0.0, 0.0, 0.0], [0.0, 0.0001, 0.0, 0.0, 0.0], [0.0, 0.0001, 0.0, 0.0, 0.0], [0.0, 0.0001, 0.0, 0.0, 0.0]]  # Cal Coefficients
        # "This is 10.30.189.0"
        n116 = Unbundle By Name(w367) -> ("LS DAS Config"=w352:T5)
        n117 = String To IP() -> (0:w362:u32)  [unwired: 1 in]
        n118 = Subtract(x=w362, y=u32 169786624) -> (x-y=w348:u32)
        n119 = call <vilib>:"Open Config Data.vi"("configuration file path"=path "c:/App Config.ini") -> ("error out"=w374:errorcluster, "file created?"=w372:bool, "refnum"=w375:T30)  [unwired: 8 in]
        n120 = Number To Decimal String(number=w348) -> (decimal integer string=w361:string)  [unwired: 1 in]
        n121 = case shown="False" w372 {
          tunnel: w375 -> [w405 w413]
          tunnel: w374 -> [w402 w411]
          tunnel: w352 -> [w401 w412]
          tunnel: [w400 w412] -> w349
          tunnel: [w406 w414] -> w350
          frame False {
            # "Read App Config.ini"
            n122 = call "Read Write LS DAS App Config.vi"("Error IN"=w402, "LS DAS Config"=w401, "Refnum in"=w405) -> ("Error OUT"=w403:errorcluster, "LS DAS Config OUT"=w400:T5, "Refnum out"=w404:T30)  [unwired: 6 in]
            n123 = call <vilib>:"Close Config Data.vi"("error in (no error)"=w403, "refnum"=w404) -> ("error out"=w407:errorcluster)  [unwired: 8 in, 1 out]
            n124 = call <vilib>:"Clear Errors.vi"("error in (no error)"=w407) -> ("error out"=w406:errorcluster)  [unwired: 6 in]
          }
          frame True {
            # "Doesn't exist, so create."
            n125 = call "Read Write LS DAS App Config.vi"("Write (F)"=TRUE, "Error IN"=w411, "LS DAS Config"=w412, "Refnum in"=w413) -> ("Error OUT"=w410:errorcluster, "Refnum out"=w408:T30)  [unwired: 5 in, 1 out]
            n126 = call <vilib>:"Close Config Data.vi"("error in (no error)"=w410, "refnum"=w408) -> ("error out"=w414:errorcluster)  [unwired: 8 in, 1 out]
          }
        }
        n127 = Concatenate Strings("/c/" ("string"), w361, ".cal" ("string")) -> (w353:string)
        n128 = String To Path(string=w353) -> (path=w354:path)
        n129 = To Long Integer(number=w348) -> (32bit integer=w347:i32)
        n130 = Bundle By Name(cluster=w349, "Data Log Init.IP Last 3"=w347) -> (w334:T5)
        n131 = Unbundle By Name(w334) -> ("Bank 1 Offset"=w339:dbl, "Bank 2 Offset"=w338:dbl, "Bank2 Record Rate"=w331:u16)
        n132 = local write "Bank 1 Voltage Offset:"(w339) -> ()
        n133 = local write "Bank 2 Voltage Offset:"(w338) -> ()
        n134 = call "Get Elapsed Times.vi"("Error In"=w350, "Path"=path "c:/ElapsedTimes" ("file (use dialog)")) -> ("Error Out"=w356:errorcluster, "Elapsed Times"=w368:dbl[])  [unwired: 8 in]
        n135 = call <vilib>:"Clear Errors.vi"("error in (no error)"=w356) -> ("error out"=w357:errorcluster)  [unwired: 6 in]
        n136 = Equal?(x=w331, y=enum16{"4.37", "1000"}."4.37" ("Bank 2 Record Rate (hz)")) -> (x = y?=w330:bool)
        n137 = call "Get Pressure Offsets.vi"("Error In"=w357, "Path"=path "c:/PressureOffsets" ("file (use dialog)")) -> ("Error Out"=w355:errorcluster, "Pressure Offsets"=w369:dbl[])  [unwired: 8 in]
        n138 = call <vilib>:"Clear Errors.vi"("error in (no error)"=w355) -> ("error out"=w345:errorcluster)  [unwired: 6 in]
        n139 = call "Get Initial LS Data.vi"("Error In"=w345, "Path"=path "c:/Monitored Statistics") -> ("Error Out"=w344:errorcluster, "Initial LS Data"=w337:T8)  [unwired: 8 in]
        n140 = call <vilib>:"Clear Errors.vi"("error in (no error)"=w344) -> ("error out"=w343:errorcluster)  [unwired: 6 in]
        n141 = call "Get Cal Coefficients.vi"("Error In"=w343, "Path"=w354) -> ("Error"=w364:bool, "Cal Coefficients"=w365:dbl[][])  [unwired: 7 in, 1 out]
        n142 = case shown="False" w364 {
          tunnel: w365 -> [_ w379]
          tunnel: [w376 w378] -> w351
          tunnel: w358 -> [w376 w377]
          frame True {
          }
          frame False {
            n143 = for {
              tunnel: w379 -> [w381] mode=indexing
              shift-right: [w382] -> w378
              shift-left: w377 -> [w383]
              i -> [w380]
              n144 = Index Array(array=w381) -> (element #1=w394:dbl, element #2=w393:dbl, element #3=w392:dbl, element #4=w388:dbl, element #5=w387:dbl)  [unwired: 5 in]
              n145 = Equal To 0?(x=w394) -> (x = 0?=w391:bool)
              n146 = Equal To 0?(x=w393) -> (x = 0?=w390:bool)
              n147 = Equal To 0?(x=w392) -> (x = 0?=w389:bool)
              n148 = Equal To 0?(x=w388) -> (x = 0?=w386:bool)
              n149 = Equal To 0?(x=w387) -> (x = 0?=w385:bool)
              n150 = Compound Arithmetic op=AND(w391, w390, w389, w386, w385) -> (w384:bool)
              n151 = case shown="False" w384 {
                tunnel: w383 -> [w398 w399]
                tunnel: [w397 w399] -> w382
                tunnel: w381 -> [w396 _]
                tunnel: w380 -> [w395 _]
                frame False {
                  n152 = Replace Array Subset(array=w398, new element=w396, index (row)=w395) -> (w397:dbl[][])  [unwired: 1 in]
                }
                frame True {
                }
              }
            }
          }
        }
        n153 = Get Volume Info(11:path "u:/" ("path")) -> (2:w336:i64)  [unwired: 1 in, 5 out]
        n154 = call "Handle Profile Resume Info.vi"("Read(F)/Write(T)"=FALSE) -> ("Current Step Out"=w342:i32, "Step Time Left Out"=w341:dbl)  [unwired: 13 in]
        n155 = Bundle By Name(cluster=w367, "LS DAS Config"=w334, "Initial Times"=w368, "Pressure Offsets"=w369, "CalArray"=w351, "Initial LS Data"=w337, "Current Step"=w342, "Step Time Left"=w341) -> (w366:T23)
        n156 = local write "Step:"(w342) -> ()
        n157 = local write "Time Left:"(w341) -> ()
        n158 = call "LS DAS Global.vi"("Bank2Slow In"=w330, "Mode"=T25."Write Init Data", "Initial LS Data In"=w337, "SDmax'"=w336) -> ()  [unwired: 5 in, 7 out]
      }
      frame "Init" {
        w433 = TRUE ("Visible")
        w426 = T28."Enabled" ("Disabled")
        w436 = u16 0 items=["0 - Off", "1 - On", "2 - Pulsing"] ("Bank 1 Power State:")
        w421 = FALSE ("Running?")
        w454 = T7[] [enum."Get Profiles", enum."Enable Background", enum."Get/Release Control", enum."Update Controls", enum."Stop Profile"] items=["Main", "Init Files", "Init", "Unused", "Save As", "Start Profile", "Check Step Time", "Alarm", "Alarm Dismiss", "Run Step", "Stop Profile", "Cycle Reset", "Time Reset", "Time Reset All", "Time Set", "Tare CTs", "Save Profile", "Open Profile", "Get Profiles", "Update Screen", "Update Controls", "Save App Config", "Write Outputs", "Disable Background", "Enable Background", "Get/Release Control", "Log Fuel Change", "Fuel Change Popup", "Read Inputs", "Remote Timer Reset", "Controller Change", "Get Alarms", "Init Alarms", "Save Alarms", "Voltage Selection", "Set Watlow Temp 1", "Set Watlow Temp 2", "Get Pressure", "Write Tare Pressure", "Adjust Controls", "Reinit ADC", "Write Initial Times", "Write Pumps Present", "HMI Command", "Save Pump Times", "Check Pump Stop Time", "Save LS App Config", "Init Data File", "Reset LS Cycles", "Reset Anomalies", "Reset Opens", "Save LS Data", "Save LS Test Data", "Check Serial Numbers", "Main Tab", "Allow Data Note", "Resume Profile", "Pause Profile", "Allow Pause Note", "Clear Graph"]
        # "This solves an issue where location wouldn't\nshow up in the built version."
        n159 = Unbundle By Name(w460) -> ("LS DAS Config.Profiles Path"=w457:path, "LS DAS Config.Location"=w458:string, "LS DAS Config.Serial Numbers"=w420:string[], "LS DAS Config.CA Number"=w434:string, "LS DAS Config.Data File Name"=w425:string)
        "Location:" <- w458
        n160 = call "Init DAS FPGA.vi"("FPGA Ref"=w417) -> ("error out"=w416:errorcluster)  [unwired: 9 in, 1 out]
        n161 = flat-sequence {
          tunnel: w459 -> [w483]
          tunnel: w416 -> [_]
          frame #0 {
            n162 = Set Occurrence(w483) -> ()
          }
        }
        n163 = property on="Replace SD Card" class="Bool (strict)"("Visible"=FALSE) -> ()  [unwired: 2 in, 2 out]
        n164 = local write "Main Tab"(T27."Main" ("Main Tab")) -> ()
        n165 = local write "pb.Run Profile"(FALSE ("pb.Run Profile")) -> ()
        n166 = local write "Bank 1 Power State:"(w436) -> ()
        n167 = local write "Bank 2 Power State:"(w436) -> ()
        n168 = property on="Location:" class="Str"("Text.Text"=w458) -> ()  [unwired: 2 in, 2 out]
        n169 = Empty String/Path?(string/path=w434) -> (empty?=w427:bool)
        n170 = Empty String/Path?(string/path=w425) -> (empty?=w435:bool)
        n171 = call <vilib>:"Check if File or Folder Exists.vi"("path"=path "u:/CA Numbers" ("base path")) -> ("error out"=w449:errorcluster, "file or folder exists?"=w451:bool, "dup path"=w450:path)  [unwired: 8 in]
        n172 = Or(x=w427, y=w435) -> (x .or. y?=w432:bool)
        n173 = case shown="False" w451 {
          tunnel: w450 -> [w480 w482]
          tunnel: w449 -> [w479 w481]
          tunnel: [w478 w482] -> w447
          tunnel: [w477 w481] -> w442
          frame False {
            n174 = Create Folder(path (use dialog)=w480, error in=w479) -> (created path=w478:path, error out=w477:errorcluster)  [unwired: 1 in, 1 out]
          }
          frame True {
          }
        }
        n175 = call <vilib>:"Check if File or Folder Exists.vi"("path"=w457) -> ("file or folder exists?"=w464:bool, "dup path"=w463:path)  [unwired: 8 in, 1 out]
        n176 = Build Path(base path=w447, name or relative path=w434) -> (appended path=w444:path)
        n177 = case shown="False" w464 {
          tunnel: w463 -> [w484 _]
          frame False {
            n178 = Create Folder(path (use dialog)=w484) -> ()  [unwired: 2 in, 3 out]
          }
          frame True {
          }
        }
        n179 = call <vilib>:"Check if File or Folder Exists.vi"("error in (no error)"=w442, "path"=w444) -> ("error out"=w446:errorcluster, "file or folder exists?"=w428:bool, "dup path"=w445:path)  [unwired: 7 in]
        n180 = Or(x=w428, y=w427) -> (x .or. y?=w429:bool)
        n181 = case shown="False" w429 {
          tunnel: w445 -> [w474 w476]
          tunnel: w446 -> [w473 w475]
          tunnel: [w472 w476] -> w443
          tunnel: [w471 w475] -> w438
          frame False {
            n182 = Create Folder(path (use dialog)=w474, error in=w473) -> (created path=w472:path, error out=w471:errorcluster)  [unwired: 1 in, 1 out]
          }
          frame True {
          }
        }
        n183 = Build Path(base path=w443, name or relative path=w425) -> (appended path=w439:path)
        n184 = property on="Data File Name:" class="Str"("Visible"=w433, "DisabledEnum"=w426) -> ()  [unwired: 2 in, 2 out]
        n185 = call <vilib>:"Check if File or Folder Exists.vi"("error in (no error)"=w438, "path"=w439) -> ("error out"=w440:errorcluster, "file or folder exists?"=w431:bool, "dup path"=w441:path)  [unwired: 7 in]
        n186 = Or(x=w431, y=w432) -> (x .or. y?=w430:bool)
        n187 = case shown="False" w430 {
          tunnel: w441 -> [w468 w470]
          tunnel: w440 -> [w467 w469]
          tunnel: [w465 w470] -> w419
          tunnel: [w466 w469] -> w437
          frame False {
            n188 = Create Folder(path (use dialog)=w468, error in=w467) -> (created path=w465:path, error out=w466:errorcluster)  [unwired: 1 in, 1 out]
          }
          frame True {
          }
        }
        n189 = property on="pb.Run Profile" class="Bool (strict)"("Visible"=w433, "DisabledEnum"=w426) -> ()  [unwired: 2 in, 2 out]
        n190 = call <vilib>:"Clear Errors.vi"("error in (no error)"=w437) -> ()  [unwired: 6 in, 1 out]
        n191 = Bundle(cluster=T26 {"Running?"=FALSE, "Record"=FALSE, "Data Filepath"=path "", "Serial Numbers"=[]} ("LS Cluster In"), "Running?"=w421, "Record"=w421, "Data Filepath"=w419, "Serial Numbers"=w420) -> (w423:T26)
        n192 = call "LS DAS Global.vi"("Mode"=T25."Main Writes", "LS Cluster In"=w423) -> ()  [unwired: 7 in, 7 out]
        n193 = Bundle By Name(cluster=w460, "pb.Run Profile"=w421, "LS Data Filepath"=w419, "Record Step"=FALSE) -> (w461:T23)
        n194 = Insert Into Array(array=w455, index=0, new element=w454) -> (w452:T7[])
      }
      frame "Unused" {
        "Replace SD Card" <- TRUE ("Replace SD Card")
      }
      frame "Get Profiles" {
        n195 = Unbundle By Name(w495) -> ("LS DAS Config.Profiles Path"=w496:path)
        n196 = List Folder(path=w496) -> (filenames=w493:string[], error out=w492:errorcluster)  [unwired: 3 in, 2 out]
        n197 = call <vilib>:"Clear Errors.vi"("error in (no error)"=w492) -> ()  [unwired: 6 in, 1 out]
        n198 = property on="Profile Name:" class="CmbBox"("Strings[]"=w493) -> ()  [unwired: 2 in, 2 out]
        n199 = Bundle By Name(cluster=w495, "Profiles"=w493) -> (w494:T23)
        n200 = Insert Into Array(array=w489, index=0, new element=Sequence_States."Open Profile") -> (w488:T7[])
      }
      frame "Open Profile" {
        w498 = T7[] [enum."Update Screen", enum."Save App Config"] items=["Main", "Init Files", "Init", "Unused", "Save As", "Start Profile", "Check Step Time", "Alarm", "Alarm Dismiss", "Run Step", "Stop Profile", "Cycle Reset", "Time Reset", "Time Reset All", "Time Set", "Tare CTs", "Save Profile", "Open Profile", "Get Profiles", "Update Screen", "Update Controls", "Save App Config", "Write Outputs", "Disable Background", "Enable Background", "Get/Release Control", "Log Fuel Change", "Fuel Change Popup", "Read Inputs", "Remote Timer Reset", "Controller Change", "Get Alarms", "Init Alarms", "Save Alarms", "Voltage Selection", "Set Watlow Temp 1", "Set Watlow Temp 2", "Get Pressure", "Write Tare Pressure", "Adjust Controls", "Reinit ADC", "Write Initial Times", "Write Pumps Present", "HMI Command", "Save Pump Times", "Check Pump Stop Time", "Save LS App Config", "Init Data File", "Reset LS Cycles", "Reset Anomalies", "Reset Opens", "Save LS Data", "Save LS Test Data", "Check Serial Numbers", "Main Tab", "Allow Data Note", "Resume Profile", "Pause Profile", "Allow Pause Note", "Clear Graph"]
        n201 = Unbundle By Name(w510) -> ("LS DAS Config.Profiles Path"=w512:path, "LS DAS Config.Current Profile"=w511:string)
        n202 = Build Path(base path=w512, name or relative path=w511) -> (appended path=w507:path)
        n203 = Read from Text File(file (use dialog)=w507) -> (refnum out=w505:refnum<file>, text=w506:string, error out=w504:errorcluster)  [unwired: 3 in, 1 out]
        n204 = Close File(refnum=w505, error in=w504) -> (error out=w503:errorcluster)  [unwired: 1 out]
        n205 = case shown="No Error" w503 {
          tunnel: w506 -> [w514 _]
          tunnel: [w515 string[][] []] -> w497
          frame No Error {
            n206 = Spreadsheet String To Array(delimiter (Tab)=",", format string="%s", spreadsheet string=w514, array type (2D Dbl)=string[][] []) -> (array=w515:string[][])
          }
          frame Error {
          }
        }
        n207 = Array Size(array=w497) -> (size(s)=w508:i32[])
        n208 = Index Array(array=w508) -> (element=w502:i32)  [unwired: 1 in]
        n209 = Bundle By Name(cluster=w510, "Profile"=w497, "# of Steps"=w502) -> (w509:T23)
        n210 = Insert Into Array(array=w500, index=0, new element=w498) -> (w499:T7[])
      }
      frame "Save Profile" {
        n211 = Unbundle By Name(w524) -> ("LS DAS Config.Profiles Path"=w528:path, "LS DAS Config.Current Profile"=w526:string, "Profile"=w527:string[][])
        n212 = Empty String/Path?(string/path=w526) -> (empty?=w525:bool)
        n213 = case shown="False" w525 {
          tunnel: w528 -> [w532 _]
          tunnel: w526 -> [w531 _]
          tunnel: w527 -> [w530 _]
          tunnel: [w529 string[][] [] ("Profile OUT")] -> w521
          frame False {
            n214 = call "Save Profile.vi"("Profile"=w530, "Current Profile"=w531, "Profiles Path"=w532) -> ("Profile OUT"=w529:string[][])  [unwired: 8 in]
          }
          frame True {
          }
        }
        n215 = Array Size(array=w521) -> (size(s)=w522:i32[])
        n216 = Index Array(array=w522) -> (element=w520:i32)  [unwired: 1 in]
        n217 = Bundle By Name(cluster=w524, "Profile"=w521, "# of Steps"=w520) -> (w523:T23)
      }
      frame "Start Profile" {
        w540 = TRUE ("Running?")
        w544 = T7[] [enum."Check Step Time"] items=["Main", "Init Files", "Init", "Unused", "Save As", "Start Profile", "Check Step Time", "Alarm", "Alarm Dismiss", "Run Step", "Stop Profile", "Cycle Reset", "Time Reset", "Time Reset All", "Time Set", "Tare CTs", "Save Profile", "Open Profile", "Get Profiles", "Update Screen", "Update Controls", "Save App Config", "Write Outputs", "Disable Background", "Enable Background", "Get/Release Control", "Log Fuel Change", "Fuel Change Popup", "Read Inputs", "Remote Timer Reset", "Controller Change", "Get Alarms", "Init Alarms", "Save Alarms", "Voltage Selection", "Set Watlow Temp 1", "Set Watlow Temp 2", "Get Pressure", "Write Tare Pressure", "Adjust Controls", "Reinit ADC", "Write Initial Times", "Write Pumps Present", "HMI Command", "Save Pump Times", "Check Pump Stop Time", "Save LS App Config", "Init Data File", "Reset LS Cycles", "Reset Anomalies", "Reset Opens", "Save LS Data", "Save LS Test Data", "Check Serial Numbers", "Main Tab", "Allow Data Note", "Resume Profile", "Pause Profile", "Allow Pause Note", "Clear Graph"]
        w547 = 0 ("Current Step")
        w542 = T28."Disabled" ("Disabled")
        # "havent yet seen if first step is to be recorded"
        n218 = Unbundle By Name(w541) -> ("LS Data Filepath"=w536:path, "LS DAS Config.Serial Numbers"=w537:string[])
        n219 = Bundle(cluster=T26 {"Running?"=FALSE, "Record"=FALSE, "Data Filepath"=path "", "Serial Numbers"=[]} ("LS Cluster In"), "Running?"=w540, "Record"=FALSE ("Running?"), "Data Filepath"=w536, "Serial Numbers"=w537) -> (w539:T26)
        n220 = call "LS DAS Global.vi"("Mode"=T25."Main Writes", "LS Cluster In"=w539) -> ()  [unwired: 7 in, 7 out]
        n221 = property on="Bank 1" class="Clust (strict)"("DisabledEnum"=w542) -> ()  [unwired: 2 in, 2 out]
        n222 = property on="Bank 2" class="Clust (strict)"("DisabledEnum"=w542) -> ()  [unwired: 2 in, 2 out]
        n223 = property on="Live Data Tab" class="TabCtl (strict)"("DisabledEnum"=w542) -> ()  [unwired: 2 in, 2 out]
        n224 = property on="Pump Timers Tab" class="TabCtl (strict)"("DisabledEnum"=w542) -> ()  [unwired: 2 in, 2 out]
        n225 = Get Date/Time In Seconds() -> (seconds since 1Jan1904=w550:timestamp)
        n226 = To Double Precision Float(number=w550) -> (double precision float=w549:dbl)
        n227 = Bundle By Name(cluster=w541, "Run Profile"=TRUE, "Step Start Time"=w549, "Last Profile Time"=w549, "Step Time"=0.0, "Current Step"=w547, "Stagger Counter"=w547, "pb.Run Profile"=w540) -> (w552:T23)
        n228 = Insert Into Array(array=w546, index=0, new element=w544) -> (w545:T7[])
      }
      frame "Check Step Time" {
        w556 = 10 ("y")
        # "Time elapsed since\nstart of step."
        n229 = Unbundle By Name(w584) -> ("ProfileMinute"=w559:i32, "Step Start Time"=w586:dbl, "Step Time"=w585:dbl, "Current Step"=w582:i32, "LS DAS Config.Stagger Time (ms)"=w567:i32, "Stagger Counter"=w573:i32)
        n230 = Get Date/Time In Seconds() -> (seconds since 1Jan1904=w562:timestamp)
        n231 = Increment(x=w573) -> (x+1=w568:i32)
        n232 = To Double Precision Float(number=w562) -> (double precision float=w581:dbl)
        n233 = Multiply(x=w567, y=w568) -> (x*y=w579:i32)
        n234 = Subtract(x=w581, y=w586) -> (x-y=w578:dbl)
        n235 = Seconds To Date/Time(time stamp (now)=w562) -> (date time rec=w561:T31)  [unwired: 1 in]
        n236 = To Double Precision Float(number=w579) -> (double precision float=w572:dbl)
        n237 = Unbundle By Name(w561) -> ("minute"=w558:i32)
        n238 = Divide(x=w572, y=1000.0) -> (x/y=w570:dbl)
        n239 = Not Equal To 0?(x=w567) -> (x != 0?=w566:bool)
        n240 = Greater Or Equal?(x=w578, y=w570) -> (x >= y?=w577:bool)
        n241 = Less Or Equal?(x=w573, y=4) -> (x <= y?=w575:bool)
        n242 = Subtract(x=w585, y=w578) -> (x-y=w563:dbl)
        n243 = Compound Arithmetic op=AND(w577, w575, w566) -> (w574:bool)
        n244 = Less Or Equal To 0?(x=w563) -> (x <= 0?=w569:bool)
        n245 = Quotient & Remainder(x=w559, y=w556) -> (floor(x/y)=w554:i32)  [unwired: 1 out]
        n246 = Quotient & Remainder(x=w558, y=w556) -> (floor(x/y)=w555:i32)  [unwired: 1 out]
        n247 = case shown="False" w569 {
          tunnel: [w596 w604] -> w557
          tunnel: w582 -> [w597 w606]
          tunnel: [w597 w605] -> w564
          tunnel: [w593 0 ("Stagger Counter")] -> w580
          tunnel: w574 -> [w595 _]
          tunnel: w573 -> [w594 _]
          tunnel: w565 -> [w592 _]
          frame False {
            # "There's time left.  Update screen."
            n248 = case shown="True" w595 {
              tunnel: [w598 w602] -> w596
              tunnel: w594 -> [w599 w601]
              tunnel: [w599 w600] -> w593
              tunnel: w592 -> [w598 _]
              frame False {
              }
              frame True {
                w602 = T7[] [enum."Run Step"] items=["Main", "Init Files", "Init", "Unused", "Save As", "Start Profile", "Check Step Time", "Alarm", "Alarm Dismiss", "Run Step", "Stop Profile", "Cycle Reset", "Time Reset", "Time Reset All", "Time Set", "Tare CTs", "Save Profile", "Open Profile", "Get Profiles", "Update Screen", "Update Controls", "Save App Config", "Write Outputs", "Disable Background", "Enable Background", "Get/Release Control", "Log Fuel Change", "Fuel Change Popup", "Read Inputs", "Remote Timer Reset", "Controller Change", "Get Alarms", "Init Alarms", "Save Alarms", "Voltage Selection", "Set Watlow Temp 1", "Set Watlow Temp 2", "Get Pressure", "Write Tare Pressure", "Adjust Controls", "Reinit ADC", "Write Initial Times", "Write Pumps Present", "HMI Command", "Save Pump Times", "Check Pump Stop Time", "Save LS App Config", "Init Data File", "Reset LS Cycles", "Reset Anomalies", "Reset Opens", "Save LS Data", "Save LS Test Data", "Check Serial Numbers", "Main Tab", "Allow Data Note", "Resume Profile", "Pause Profile", "Allow Pause Note", "Clear Graph"]
                n249 = Increment(x=w601) -> (x+1=w600:i32)
              }
            }
          }
          frame True {
            w604 = T7[] [enum."Run Step"] items=["Main", "Init Files", "Init", "Unused", "Save As", "Start Profile", "Check Step Time", "Alarm", "Alarm Dismiss", "Run Step", "Stop Profile", "Cycle Reset", "Time Reset", "Time Reset All", "Time Set", "Tare CTs", "Save Profile", "Open Profile", "Get Profiles", "Update Screen", "Update Controls", "Save App Config", "Write Outputs", "Disable Background", "Enable Background", "Get/Release Control", "Log Fuel Change", "Fuel Change Popup", "Read Inputs", "Remote Timer Reset", "Controller Change", "Get Alarms", "Init Alarms", "Save Alarms", "Voltage Selection", "Set Watlow Temp 1", "Set Watlow Temp 2", "Get Pressure", "Write Tare Pressure", "Adjust Controls", "Reinit ADC", "Write Initial Times", "Write Pumps Present", "HMI Command", "Save Pump Times", "Check Pump Stop Time", "Save LS App Config", "Init Data File", "Reset LS Cycles", "Reset Anomalies", "Reset Opens", "Save LS Data", "Save LS Test Data", "Check Serial Numbers", "Main Tab", "Allow Data Note", "Resume Profile", "Pause Profile", "Allow Pause Note", "Clear Graph"]
            # "No time left.  Go to next step."
            n250 = Increment(x=w606) -> (x+1=w605:i32)
          }
        }
        n251 = Not Equal?(x=w554, y=w555) -> (x != y?=w560:bool)
        n252 = case shown="True" w560 {
          tunnel: w557 -> [w587 w591]
          tunnel: [w587 w590] -> w553
          frame False {
          }
          frame True {
            n253 = Insert Into Array(array=w591, index=0, new element=Sequence_States."Save LS Data") -> (w590:T7[])
          }
        }
        n254 = Bundle By Name(cluster=w584, "ProfileMinute"=w558, "Last Profile Time"=w581, "Step Time Left"=w563, "New Step"=w569, "Current Step"=w564, "Stagger Counter"=w580) -> (w583:T23)
      }
      frame "Run Step" {
        w624 = T7[] [enum."Write Outputs", enum."Read Inputs", enum."Update Screen"] items=["Main", "Init Files", "Init", "Unused", "Save As", "Start Profile", "Check Step Time", "Alarm", "Alarm Dismiss", "Run Step", "Stop Profile", "Cycle Reset", "Time Reset", "Time Reset All", "Time Set", "Tare CTs", "Save Profile", "Open Profile", "Get Profiles", "Update Screen", "Update Controls", "Save App Config", "Write Outputs", "Disable Background", "Enable Background", "Get/Release Control", "Log Fuel Change", "Fuel Change Popup", "Read Inputs", "Remote Timer Reset", "Controller Change", "Get Alarms", "Init Alarms", "Save Alarms", "Voltage Selection", "Set Watlow Temp 1", "Set Watlow Temp 2", "Get Pressure", "Write Tare Pressure", "Adjust Controls", "Reinit ADC", "Write Initial Times", "Write Pumps Present", "HMI Command", "Save Pump Times", "Check Pump Stop Time", "Save LS App Config", "Init Data File", "Reset LS Cycles", "Reset Anomalies", "Reset Opens", "Save LS Data", "Save LS Test Data", "Check Serial Numbers", "Main Tab", "Allow Data Note", "Resume Profile", "Pause Profile", "Allow Pause Note", "Clear Graph"]
        n255 = Unbundle By Name(w618) -> ("Profile"=w636:string[][], "Current Step"=w635:i32, "# of Steps"=w634:i32, "LS DAS Config.Cycles Completed"=w633:u32, "LS DAS Config.Pumps Present"=w625:T22, "New Step"=w640:bool, "Step Start Time"=w639:dbl, "Run Profile"=w614:bool, "LS DAS Config.Profile Record"=w610:bool, "LS Data Filepath"=w612:path, "LS DAS Config.Serial Numbers"=w613:string[])
        n256 = call "Run Step.vi"("Profile"=w636, "Current Step in"=w635, "# of Steps"=w634, "Cycles Completed in"=w633, "Pumps Present"=w625) -> ("Bank1State"=w622:u16, "Bank2State"=w621:u16, "Record"=w609:bool, "LS Freq"=w620:dbl, "LS Duty"=w619:dbl, "PS Cmd"=w632:dbl, "Press Cmd"=w631:dbl, "Ignition Relays"=w630:T22, "Current Step out"=w629:i32, "Cycles Completed out"=w628:u32, "Step Time"=w627:dbl, "Controller CMDs"=w626:dbl[], "Power Relays"=w617:T22)  [unwired: 10 in]
        n257 = And(x=w609, y=w610) -> (x .and. y?=w608:bool)
        n258 = Bundle(cluster=T26 {"Running?"=FALSE, "Record"=FALSE, "Data Filepath"=path "", "Serial Numbers"=[]} ("LS Cluster In"), "Running?"=w614, "Record"=w608, "Data Filepath"=w612, "Serial Numbers"=w613) -> (w611:T26)
        n259 = call "LS DAS Global.vi"("Mode"=T25."Main Writes", "LS Cluster In"=w611) -> ()  [unwired: 7 in, 7 out]
        n260 = local write "Bank 1 Power State:"(w622) -> ()
        n261 = local write "Bank 2 Power State:"(w621) -> ()
        n262 = local write "LS Cycle Time (ms):"(w620) -> ()
        n263 = local write "LS On Time (ms):"(w619) -> ()
        n264 = case shown="False" w640 {
          tunnel: [w645 w646] -> w623
          tunnel: w639 -> [w645 _]
          tunnel: w626 -> [_ _]
          frame False {
          }
          frame True {
            n265 = Get Date/Time In Seconds() -> (seconds since 1Jan1904=w647:timestamp)
            n266 = To Double Precision Float(number=w647) -> (double precision float=w646:dbl)
          }
        }
        n267 = Insert Into Array(array=w637, index=0, new element=w624) -> (w616:T7[])
        n268 = flat-sequence {
          tunnel: w623 -> [_]
          frame #0 {
            n269 = Tick Count (ms)() -> (millisecond timer value=w644:u32)
            n270 = feedback #1() -> (w643:u32)  [unwired: 1 in]
            n271 = feedback-in #1(w644) -> ()
            n272 = Subtract(x=w644, y=w643) -> (x-y=→"Run Step (ms)":u32)
          }
        }
        n273 = Bundle By Name(cluster=w618, "Bank 1 State:"=w622, "Bank 2 State:"=w621, "LS DAS Config.LS Power (Freq):"=w620, "LS DAS Config.LS Power (Duty):"=w619, "Tank CMDs.PS CMD"=w632, "Tank CMDs.Press CMD"=w631, "Ignition Relay"=w630, "Current Step"=w629, "LS DAS Config.Cycles Completed"=w628, "Step Time"=w627, "Controller CMDs"=w626, "Power Relay"=w617, "Step Start Time"=w623, "Record Step"=w609) -> (w641:T23)
      }
      frame "Write Outputs" {
        w652 = 40000.0 ("x")
        # "T:Anomalies     F:Opens"
        n274 = Unbundle By Name(w649) -> ("LS DAS Config.Bank 1 Present"=w676:T2, "LS DAS Config.Bank 2 Present"=w675:T29, "LS DAS Config.Detection Mode"=w661:i32, "Bank 1 State:"=w668:u16, "Bank 2 State:"=w671:u16, "LS DAS Config.LS Power (Freq):"=w654:dbl, "LS DAS Config.LS Power (Duty):"=w670:dbl, "LS DAS Config.Bank 1 Offset"=w651:dbl, "LS DAS Config.Bank 2 Offset"=w650:dbl)
        n275 = Cluster To Array(cluster=w676) -> (array=w664:bool[])
        n276 = Cluster To Array(cluster=w675) -> (array=w666:bool[])
        n277 = Equal To 0?(x=w661) -> (x = 0?=w660:bool)
        n278 = Multiply(x=w652, y=w654) -> (x*y=w653:dbl)
        n279 = case shown="2" w668 {
          tunnel: [FALSE FALSE TRUE] -> w667
          tunnel: [FALSE TRUE FALSE] -> w656
          frame 0, Default {
            # "Off"
          }
          frame 1 {
            # "On"
          }
          frame 2 {
            # "Pulsing"
          }
        }
        n280 = case shown="2" w671 {
          tunnel: [FALSE FALSE TRUE] -> w669
          tunnel: [FALSE TRUE FALSE] -> w657
          frame 0, Default {
            # "Off"
          }
          frame 1 {
            # "On"
          }
          frame 2 {
            # "Pulsing"
          }
        }
        n281 = Multiply(x=w652, y=w670) -> (x*y=w674:dbl)
        n282 = To Unsigned Long Integer(number=w653) -> (unsigned 32bit integer=w672:u32)
        n283 = To Long Integer(number=w674) -> (32bit integer=w673:i32)
        n284 = Insert Into Array(array=w666, index=0, new element=w664) -> (w663:bool[])
        n285 = Not(x=w660) -> (.not. x?=w659:bool)
        n286 = And(x=w663, y=w660) -> (x .and. y?=w662:bool[])
        n287 = And(x=w663, y=w659) -> (x .and. y?=w658:bool[])
        n288 = xnode "Read/Write Control"("FPGA VI Reference In"=w655, "Enable Readings"=w663, "Enable Cycles"=w662, "Enable Opens"=w658, "Bank1(Pulse/Const)"=w667, "Bank1Const(On/Off)"=w656, "Bank2(Pulse/Const)"=w669, "Bank2Const(On/Off)"=w657, "PWM Period (Ticks)"=w672, "Duty (Ticks)"=w673, "B1offset"=w651, "B2offset"=w650) -> ()  [unwired: 1 in, 2 out]
      }
      frame "Read Inputs" {
        n289 = Unbundle By Name(w696) -> ("Initial LS Data"=w690:T8)
        n290 = flat-sequence {
          frame #0 {
            n291 = Tick Count (ms)() -> (millisecond timer value=w699:u32)
            n292 = feedback #2() -> (w698:u32)  [unwired: 1 in]
            n293 = feedback-in #2(w699) -> ()
            n294 = Subtract(x=w699, y=w698) -> (x-y=→"Read Inputs (ms)":u32)
          }
        }
        n295 = Tick Count (ms)() -> (millisecond timer value=w692:u32)
        n296 = call "Get Time and Date.vi"() -> ("Time/Date"=w694:string)  [unwired: 11 in]
        n297 = call "Get LS DAS Data.vi"("Initial LS Data"=w690, "FPGA Ref"=w691) -> ("LS Data"=w689:T8)  [unwired: 9 in]
        n298 = Bundle By Name(cluster=w696, "Inputs Timer"=w692, "Time/Date"=w694, "LS Data"=w689) -> (w695:T23)
      }
      frame "Update Screen" {
        w703 = FALSE
        # "Backup current step and time left every ten run minutes and at the start of every new step"
        n299 = Unbundle By Name(w728) -> ("LS DAS Config.Cycles Completed"=→"Cycles Completed:":u32, "Current Step"=w713:i32, "Step Time Left"=w714:dbl, "Time/Date"=→"Time/Date":string, "Recording"=→"Recording":bool, "LS Data"=w725:T8, "Run Profile"=w712:bool)
        "Step:" <- w713
        "Time Left:" <- w714
        n300 = Unbundle(w725) -> ("Total Cycles"=→"Total Cycles":u32[], "Steps"=→"Steps":u32[], "Anomalies Total"=→"Anomalies Total":i32[], "Cycles"=→"Cycles":u32[], "Anomalies/Cycle"=→"Anomalies/Cycle":i32[], "Anomalies (Last Cycle)"=→"Anomalies (Last Cycle)":i32[], "Opens"=→"Opens":i32[])
        n301 = case shown="True" w712 {
          tunnel: [w747 w750] -> w710
          tunnel: w734 -> [w747 w749]
          frame False {
          }
          frame True {
            w748 = T7[] [enum."Update Controls"] items=["Main", "Init Files", "Init", "Unused", "Save As", "Start Profile", "Check Step Time", "Alarm", "Alarm Dismiss", "Run Step", "Stop Profile", "Cycle Reset", "Time Reset", "Time Reset All", "Time Set", "Tare CTs", "Save Profile", "Open Profile", "Get Profiles", "Update Screen", "Update Controls", "Save App Config", "Write Outputs", "Disable Background", "Enable Background", "Get/Release Control", "Log Fuel Change", "Fuel Change Popup", "Read Inputs", "Remote Timer Reset", "Controller Change", "Get Alarms", "Init Alarms", "Save Alarms", "Voltage Selection", "Set Watlow Temp 1", "Set Watlow Temp 2", "Get Pressure", "Write Tare Pressure", "Adjust Controls", "Reinit ADC", "Write Initial Times", "Write Pumps Present", "HMI Command", "Save Pump Times", "Check Pump Stop Time", "Save LS App Config", "Init Data File", "Reset LS Cycles", "Reset Anomalies", "Reset Opens", "Save LS Data", "Save LS Test Data", "Check Serial Numbers", "Main Tab", "Allow Data Note", "Resume Profile", "Pause Profile", "Allow Pause Note", "Clear Graph"]
            n302 = Insert Into Array(array=w749, index=0, new element=w748) -> (w750:T7[])
          }
        }
        n303 = call "App Global.vi"() -> ("CPU Usage OUT"=→"CPU Usage:":dbl, "Login OUT"=w729:bool)  [unwired: 9 in, 1 out]
        n304 = local write "Login"(w729) -> ()
        n305 = Quotient & Remainder(x=w714, y=600.0) -> (floor(x/y)=w715:dbl)  [unwired: 1 out]
        n306 = feedback #3(w715) -> (w716:dbl)
        n307 = feedback-in #3(w715) -> ()
        n308 = Not Equal?(x=w716, y=w715) -> (x != y?=w711:bool)
        n309 = case shown="True" w711 {
          tunnel: w714 -> [_ w742]
          tunnel: w713 -> [_ w743]
          frame False {
          }
          frame True {
            n310 = call "Handle Profile Resume Info.vi"("Read(F)/Write(T)"=TRUE ("Write(T)/Read(F)"), "Current Step In"=w743, "Step Time Left In"=w742) -> ()  [unwired: 11 in, 2 out]
          }
        }
        n311 = call "LS DAS Global.vi"() -> ("Recording Out"=→"Recording":bool, "SD%"=w707:dbl)  [unwired: 9 in, 5 out]
        "SD Card % Usage" <- w707
        n312 = flat-sequence {
          frame #0 {
            n313 = Tick Count (ms)() -> (millisecond timer value=w746:u32)
            n314 = feedback #4() -> (w745:u32)  [unwired: 1 in]
            n315 = feedback-in #4(w746) -> ()
            n316 = Subtract(x=w746, y=w745) -> (x-y=→"Update Screen (ms)":u32)
          }
        }
        n317 = Greater?(x=w707, y=75.0) -> (0:w705:bool)
        n318 = feedback #5(w703) -> (w706:bool)
        n319 = feedback-in #5(w705) -> ()
        n320 = Greater?(x=w706, y=w703) -> (0:w701:bool)
        n321 = Less?(x=w706, y=w703) -> (x < y?=w704:bool)
        n322 = Or(x=w701, y=w704) -> (x .or. y?=w702:bool)
        n323 = Tick Count (ms)() -> (millisecond timer value=w726:u32)
        n324 = case shown="True" w702 {
          tunnel: w701 -> [_ w735]
          frame False {
          }
          frame True {
            n325 = property on="Replace SD Card" class="Bool (strict)"("Visible"=w735) -> ()  [unwired: 2 in, 2 out]
          }
        }
        n326 = case shown="True" w711 {
          tunnel: [w736 w739] -> w709
          tunnel: w710 -> [w736 w738]
          frame False {
          }
          frame True {
            w737 = T7[] [enum."Save LS Data"] items=["Main", "Init Files", "Init", "Unused", "Save As", "Start Profile", "Check Step Time", "Alarm", "Alarm Dismiss", "Run Step", "Stop Profile", "Cycle Reset", "Time Reset", "Time Reset All", "Time Set", "Tare CTs", "Save Profile", "Open Profile", "Get Profiles", "Update Screen", "Update Controls", "Save App Config", "Write Outputs", "Disable Background", "Enable Background", "Get/Release Control", "Log Fuel Change", "Fuel Change Popup", "Read Inputs", "Remote Timer Reset", "Controller Change", "Get Alarms", "Init Alarms", "Save Alarms", "Voltage Selection", "Set Watlow Temp 1", "Set Watlow Temp 2", "Get Pressure", "Write Tare Pressure", "Adjust Controls", "Reinit ADC", "Write Initial Times", "Write Pumps Present", "HMI Command", "Save Pump Times", "Check Pump Stop Time", "Save LS App Config", "Init Data File", "Reset LS Cycles", "Reset Anomalies", "Reset Opens", "Save LS Data", "Save LS Test Data", "Check Serial Numbers", "Main Tab", "Allow Data Note", "Resume Profile", "Pause Profile", "Allow Pause Note", "Clear Graph"]
            n327 = Insert Into Array(array=w738, index=0, new element=w737) -> (w739:T7[])
          }
        }
        n328 = Bundle By Name(cluster=w728, "Screen Timer"=w726) -> (w727:T23)
      }
      frame "Update Controls" {
        n329 = Unbundle By Name(w765) -> ("Profile"=w768:string[][], "LS DAS Config.Current Profile"=w767:string, "LS DAS Config.CA Number"=w766:string, "Run Profile"=w764:bool, "Recording"=w763:bool, "LS DAS Config.LS Power (Freq):"=w756:dbl, "LS DAS Config.LS Power (Duty):"=w755:dbl, "LS DAS Config.Bank 1 Present"=w754:T2, "LS DAS Config.Bank 2 Present"=w753:T29, "LS DAS Config.Data File Name"=w757:string, "LS DAS Config.Detection Mode"=w762:i32, "LS DAS Config.Serial Numbers"=w761:string[], "Bank 1 State:"=w759:u16, "Bank 2 State:"=w758:u16)
        n330 = Array To Cluster(array=w761) -> (cluster=w760:T32)
        n331 = local write "LS Cycle Time (ms):"(w756) -> ()
        n332 = local write "LS On Time (ms):"(w755) -> ()
        n333 = local write "Bank 1"(w754) -> ()
        n334 = local write "Bank 2"(w753) -> ()
        n335 = local write "Data File Name:"(w757) -> ()
        n336 = local write "Detection Mode:"(w762) -> ()
        n337 = local write "LS Serial Numbers"(w760) -> ()
        n338 = local write "Bank 1 Power State:"(w759) -> ()
        n339 = local write "Bank 2 Power State:"(w758) -> ()
        n340 = local write "pb.Run Profile"(w764) -> ()
        n341 = local write "Recording"(w763) -> ()
        n342 = case shown="False" w764 {
          tunnel: w768 -> [w771 _]
          tunnel: w767 -> [w770 _]
          tunnel: w766 -> [w769 _]
          frame False {
            n343 = local write "Profile:"(w771) -> ()
            n344 = local write "Profile Name:"(w770) -> ()
            n345 = local write "CA Number:"(w769) -> ()
          }
          frame True {
          }
        }
      }
      frame "Stop Profile" {
        w773 = FALSE ("Running?")
        w783 = u16 0 items=["0 - Off", "1 - On", "2 - Pulsing"] ("Bank 1 Power State:")
        w782 = FALSE ("Running?")
        w787 = T7[] [enum."Write Outputs", enum."Update Controls"] items=["Main", "Init Files", "Init", "Unused", "Save As", "Start Profile", "Check Step Time", "Alarm", "Alarm Dismiss", "Run Step", "Stop Profile", "Cycle Reset", "Time Reset", "Time Reset All", "Time Set", "Tare CTs", "Save Profile", "Open Profile", "Get Profiles", "Update Screen", "Update Controls", "Save App Config", "Write Outputs", "Disable Background", "Enable Background", "Get/Release Control", "Log Fuel Change", "Fuel Change Popup", "Read Inputs", "Remote Timer Reset", "Controller Change", "Get Alarms", "Init Alarms", "Save Alarms", "Voltage Selection", "Set Watlow Temp 1", "Set Watlow Temp 2", "Get Pressure", "Write Tare Pressure", "Adjust Controls", "Reinit ADC", "Write Initial Times", "Write Pumps Present", "HMI Command", "Save Pump Times", "Check Pump Stop Time", "Save LS App Config", "Init Data File", "Reset LS Cycles", "Reset Anomalies", "Reset Opens", "Save LS Data", "Save LS Test Data", "Check Serial Numbers", "Main Tab", "Allow Data Note", "Resume Profile", "Pause Profile", "Allow Pause Note", "Clear Graph"]
        w789 = T22 {"Pump 1"=FALSE, "Pump 2"=FALSE, "Pump 3"=FALSE, "Pump 4"=FALSE, "Pump 5"=FALSE, "Pump 6"=FALSE} ("Power Relay")
        n346 = Unbundle By Name(w788) -> ("LS Data Filepath"=w776:path, "LS DAS Config.Serial Numbers"=w777:string[], "Current Step"=w780:i32, "Step Time Left"=w779:dbl, "Login"=w775:bool)
        n347 = Bundle(cluster=T26 {"Running?"=FALSE, "Record"=FALSE, "Data Filepath"=path "", "Serial Numbers"=[]} ("LS Cluster In"), "Running?"=w782, "Record"=w773, "Data Filepath"=w776, "Serial Numbers"=w777) -> (w774:T26)
        n348 = call "LS DAS Global.vi"("Mode"=T25."Main Writes", "LS Cluster In"=w774) -> ()  [unwired: 7 in, 7 out]
        n349 = call "Handle Profile Resume Info.vi"("Read(F)/Write(T)"=TRUE, "Current Step In"=w780, "Step Time Left In"=w779) -> ()  [unwired: 11 in, 2 out]
        n350 = case shown="True" w775 {
          frame False {
          }
          frame True {
            w794 = T28."Enabled" ("Disabled")
            n351 = property on="Bank 1" class="Clust (strict)"("DisabledEnum"=w794) -> ()  [unwired: 2 in, 2 out]
            n352 = property on="Bank 2" class="Clust (strict)"("DisabledEnum"=w794) -> ()  [unwired: 2 in, 2 out]
            n353 = property on="Live Data Tab" class="TabCtl (strict)"("DisabledEnum"=w794) -> ()  [unwired: 2 in, 2 out]
            n354 = property on="Pump Timers Tab" class="TabCtl (strict)"("DisabledEnum"=w794) -> ()  [unwired: 2 in, 2 out]
          }
        }
        n355 = local write "Bank 1 Power State:"(w783) -> ()
        n356 = local write "Bank 2 Power State:"(w783) -> ()
        n357 = Bundle By Name(cluster=w788, "Record Step"=w773, "pb.Run Profile"=w782, "Run Profile"=FALSE, "Power Relay"=w789, "Ignition Relay"=w789, "Tank CMDs.Press CMD"=0.0, "Recording"=FALSE, "Bank 1 State:"=w783, "Bank 2 State:"=w783) -> (w785:T23)
        n358 = Insert Into Array(array=w792, index=0, new element=w787) -> (w791:T7[])
      }
      frame "Save As" {
        n359 = property on="Save As Tab" class="TabCtl (strict)"("Visible"=TRUE) -> (error out=w799:errorcluster)  [unwired: 2 in, 1 out]
        n360 = while {
          tunnel: ["pb.Save As OK"] -> w805
          tunnel: w799 -> [_]
          stop <- w807 stop-if-true
          n361 = Wait (ms)(milliseconds to wait=u32 10) -> ()  [unwired: 1 out]
          n362 = Or(x="pb.Save As OK", y="pb.Save As Cancel") -> (x .or. y?=w807:bool)
        }
        n363 = Unbundle By Name(w803) -> ("LS DAS Config.Profiles Path"=w804:path, "Profile"=w801:string[][])
        n364 = case shown="True" w805 {
          tunnel: w804 -> [_ w815]
          tunnel: [w810 w812] -> w796
          tunnel: w803 -> [w811 w817]
          tunnel: [w811 w816] -> w802
          tunnel: w801 -> [_ w814]
          frame False {
            w810 = T7[] [enum."Enable Background"] items=["Main", "Init Files", "Init", "Unused", "Save As", "Start Profile", "Check Step Time", "Alarm", "Alarm Dismiss", "Run Step", "Stop Profile", "Cycle Reset", "Time Reset", "Time Reset All", "Time Set", "Tare CTs", "Save Profile", "Open Profile", "Get Profiles", "Update Screen", "Update Controls", "Save App Config", "Write Outputs", "Disable Background", "Enable Background", "Get/Release Control", "Log Fuel Change", "Fuel Change Popup", "Read Inputs", "Remote Timer Reset", "Controller Change", "Get Alarms", "Init Alarms", "Save Alarms", "Voltage Selection", "Set Watlow Temp 1", "Set Watlow Temp 2", "Get Pressure", "Write Tare Pressure", "Adjust Controls", "Reinit ADC", "Write Initial Times", "Write Pumps Present", "HMI Command", "Save Pump Times", "Check Pump Stop Time", "Save LS App Config", "Init Data File", "Reset LS Cycles", "Reset Anomalies", "Reset Opens", "Save LS Data", "Save LS Test Data", "Check Serial Numbers", "Main Tab", "Allow Data Note", "Resume Profile", "Pause Profile", "Allow Pause Note", "Clear Graph"]
          }
          frame True {
            w812 = T7[] [enum."Enable Background", enum."Get Profiles"] items=["Main", "Init Files", "Init", "Unused", "Save As", "Start Profile", "Check Step Time", "Alarm", "Alarm Dismiss", "Run Step", "Stop Profile", "Cycle Reset", "Time Reset", "Time Reset All", "Time Set", "Tare CTs", "Save Profile", "Open Profile", "Get Profiles", "Update Screen", "Update Controls", "Save App Config", "Write Outputs", "Disable Background", "Enable Background", "Get/Release Control", "Log Fuel Change", "Fuel Change Popup", "Read Inputs", "Remote Timer Reset", "Controller Change", "Get Alarms", "Init Alarms", "Save Alarms", "Voltage Selection", "Set Watlow Temp 1", "Set Watlow Temp 2", "Get Pressure", "Write Tare Pressure", "Adjust Controls", "Reinit ADC", "Write Initial Times", "Write Pumps Present", "HMI Command", "Save Pump Times", "Check Pump Stop Time", "Save LS App Config", "Init Data File", "Reset LS Cycles", "Reset Anomalies", "Reset Opens", "Save LS Data", "Save LS Test Data", "Check Serial Numbers", "Main Tab", "Allow Data Note", "Resume Profile", "Pause Profile", "Allow Pause Note", "Clear Graph"]
            n365 = call "Save Profile.vi"("Profile"=w814, "Current Profile"="New Profile Name:", "Profiles Path"=w815) -> ()  [unwired: 8 in, 1 out]
            n366 = Bundle By Name(cluster=w817, "LS DAS Config.Current Profile"="New Profile Name:") -> (w816:T23)
          }
        }
        n367 = Insert Into Array(array=w798, index=0, new element=w796) -> (w797:T7[])
      }
      frame "Save App Config" {
        n368 = Unbundle By Name(w826) -> ("LS DAS Config"=w821:T5)
        n369 = call <vilib>:"Open Config Data.vi"("create file if necessary (T)"=TRUE, "configuration file path"=path "c:/App Config.ini") -> ("error out"=w820:errorcluster, "refnum"=w822:T30)  [unwired: 7 in, 1 out]
        n370 = call "Read Write LS DAS App Config.vi"("Write (F)"=TRUE, "Error IN"=w820, "LS DAS Config"=w821, "Refnum in"=w822) -> ("Error OUT"=w819:errorcluster, "Refnum out"=w818:T30)  [unwired: 5 in, 1 out]
        n371 = call <vilib>:"Close Config Data.vi"("error in (no error)"=w819, "refnum"=w818) -> ()  [unwired: 8 in, 2 out]
      }
      frame "Disable Background" {
        w828 = T28."Disabled and Grayed Out" ("Disabled")
        n372 = property on="Main Tab" class="TabCtl (strict)"("DisabledEnum"=w828) -> ()  [unwired: 2 in, 2 out]
        n373 = property on="pb.Stop Profile" class="Bool"("DisabledEnum"=w828) -> ()  [unwired: 2 in, 2 out]
        n374 = property on="Title Tab" class="TabCtl (strict)"("DisabledEnum"=w828) -> ()  [unwired: 2 in, 2 out]
        n375 = property on="CPU Usage:" class="DigNum (strict)"("DisabledEnum"=w828) -> ()  [unwired: 2 in, 2 out]
        n376 = property on="Pump Timers Tab" class="TabCtl (strict)"("DisabledEnum"=w828) -> ()  [unwired: 2 in, 2 out]
        n377 = property on="Live Data Tab" class="TabCtl (strict)"("DisabledEnum"=w828) -> ()  [unwired: 2 in, 2 out]
      }
      frame "Enable Background" {
        w831 = FALSE ("Visible")
        w832 = T28."Enabled" ("Disabled")
        n378 = disable-structure shown="Enabled" {
          disable-tunnel: w834 -> [w837 w839]
          frame Disabled {
            n379 = xnode "Read/Write Control"("FPGA VI Reference In"=w837, "Timer Resets"=bool[] [FALSE, FALSE, FALSE, FALSE, FALSE, FALSE] ("array")) -> ()  [unwired: 1 in, 2 out]
          }
          frame Enabled {
            w838 = bool[] [FALSE, FALSE, FALSE, FALSE, FALSE, FALSE, FALSE, FALSE, FALSE, FALSE, FALSE, FALSE] ("Opens Resets")
            n380 = xnode "Read/Write Control"("FPGA VI Reference In"=w839, "Opens Resets"=w838, "Cycle Resets"=w838) -> ()  [unwired: 1 in, 2 out]
          }
        }
        n381 = property on="Save As Tab" class="TabCtl (strict)"("Visible"=w831) -> ()  [unwired: 2 in, 2 out]
        n382 = property on="Reset Tab" class="TabCtl (strict)"("Visible"=w831) -> ()  [unwired: 2 in, 2 out]
        n383 = property on="Set Time Tab" class="TabCtl (strict)"("Visible"=w831) -> ()  [unwired: 2 in, 2 out]
        n384 = property on="Alarm Tab" class="TabCtl (strict)"("Visible"=w831) -> ()  [unwired: 2 in, 2 out]
        n385 = property on="Note Tab" class="TabCtl (strict)"("Visible"=w831) -> ()  [unwired: 2 in, 2 out]
        n386 = property on="Main Tab" class="TabCtl (strict)"("DisabledEnum"=w832) -> ()  [unwired: 2 in, 2 out]
        n387 = property on="pb.Stop Profile" class="Bool"("DisabledEnum"=w832) -> ()  [unwired: 2 in, 2 out]
        n388 = property on="Title Tab" class="TabCtl (strict)"("DisabledEnum"=w832) -> ()  [unwired: 2 in, 2 out]
        n389 = property on="CPU Usage:" class="DigNum (strict)"("DisabledEnum"=w832) -> ()  [unwired: 2 in, 2 out]
        n390 = property on="Alarm Tab" class="TabCtl (strict)"("DisabledEnum"=w832) -> ()  [unwired: 2 in, 2 out]
        n391 = property on="Pump Timers Tab" class="TabCtl (strict)"("DisabledEnum"=w832) -> ()  [unwired: 2 in, 2 out]
        n392 = property on="Live Data Tab" class="TabCtl (strict)"("DisabledEnum"=w832) -> ()  [unwired: 2 in, 2 out]
      }
      frame "Cycle Reset".."Time Reset All", "Reset LS Cycles".."Reset Opens" {
        w852 = T7[] [enum."Enable Background"] items=["Main", "Init Files", "Init", "Unused", "Save As", "Start Profile", "Check Step Time", "Alarm", "Alarm Dismiss", "Run Step", "Stop Profile", "Cycle Reset", "Time Reset", "Time Reset All", "Time Set", "Tare CTs", "Save Profile", "Open Profile", "Get Profiles", "Update Screen", "Update Controls", "Save App Config", "Write Outputs", "Disable Background", "Enable Background", "Get/Release Control", "Log Fuel Change", "Fuel Change Popup", "Read Inputs", "Remote Timer Reset", "Controller Change", "Get Alarms", "Init Alarms", "Save Alarms", "Voltage Selection", "Set Watlow Temp 1", "Set Watlow Temp 2", "Get Pressure", "Write Tare Pressure", "Adjust Controls", "Reinit ADC", "Write Initial Times", "Write Pumps Present", "HMI Command", "Save Pump Times", "Check Pump Stop Time", "Save LS App Config", "Init Data File", "Reset LS Cycles", "Reset Anomalies", "Reset Opens", "Save LS Data", "Save LS Test Data", "Check Serial Numbers", "Main Tab", "Allow Data Note", "Resume Profile", "Pause Profile", "Allow Pause Note", "Clear Graph"]
        n393 = property on="Reset Tab" class="TabCtl (strict)"("Visible"=TRUE) -> (error out=w848:errorcluster)  [unwired: 2 in, 1 out]
        n394 = while {
          tunnel: ["pb.Reset OK"] -> w850
          tunnel: w848 -> [_]
          stop <- w879 stop-if-true
          n395 = Wait (ms)(milliseconds to wait=u32 10) -> ()  [unwired: 1 out]
          n396 = Or(x="pb.Reset Cancel", y="pb.Reset OK") -> (x .or. y?=w879:bool)
        }
        n397 = case shown="True" w850 {
          tunnel: [w858 w862] -> w847
          tunnel: w856 -> [w858 w861]
          tunnel: w857 -> [_ w860]
          tunnel: w855 -> [_ w859]
          frame False {
          }
          frame True {
            n398 = case shown="\"Reset Opens\"" w859 {
              tunnel: w861 -> [w866 w873 w877]
              tunnel: [w865 w872 w877] -> w862
              tunnel: w860 -> [w864 w871 _]
              frame "Reset LS Cycles" {
                n399 = flat-sequence {
                  tunnel: w864 -> [w868]
                  frame #0 {
                    n400 = xnode "Read/Write Control"("FPGA VI Reference In"=w868, "Cycle Resets"=bool[] [TRUE, TRUE, TRUE, TRUE, TRUE, TRUE, TRUE, TRUE, TRUE, TRUE, TRUE, TRUE] ("Opens Resets")) -> ()  [unwired: 1 in, 2 out]
                  }
                  frame #1 {
                    n401 = Wait (ms)(milliseconds to wait=u32 5) -> ()  [unwired: 1 out]
                  }
                }
                n402 = Bundle By Name(cluster=w866, "Initial LS Data.Total Cycles"=u32[] [0, 0, 0, 0, 0, 0, 0, 0, 0, 0, 0, 0]) -> (w865:T23)
              }
              frame "Reset Opens" {
                n403 = flat-sequence {
                  tunnel: w871 -> [w875]
                  frame #0 {
                    n404 = xnode "Read/Write Control"("FPGA VI Reference In"=w875, "Opens Resets"=bool[] [TRUE, TRUE, TRUE, TRUE, TRUE, TRUE, TRUE, TRUE, TRUE, TRUE, TRUE, TRUE]) -> ()  [unwired: 1 in, 2 out]
                  }
                  frame #1 {
                    n405 = Wait (ms)(milliseconds to wait=u32 5) -> ()  [unwired: 1 out]
                  }
                }
                n406 = Bundle By Name(cluster=w873, "Initial LS Data.Opens"=i32[] [0, 0, 0, 0, 0, 0, 0, 0, 0, 0, 0, 0]) -> (w872:T23)
              }
              frame Default {
              }
            }
          }
        }
        n407 = Unbundle By Name(w847) -> ("LS DAS Config.Bank2 Record Rate"=w841:u16, "Initial LS Data"=w846:T8)
        n408 = Get Volume Info(11:path "u:/" ("path")) -> (2:w844:i64)  [unwired: 1 in, 5 out]
        n409 = Equal?(x=enum16{"4.37", "1000"}."4.37" ("Bank 2 Record Rate (hz)"), y=w841) -> (x = y?=w840:bool)
        n410 = call "LS DAS Global.vi"("Bank2Slow In"=w840, "Mode"=T25."Write Init Data", "Initial LS Data In"=w846, "SDmax'"=w844) -> ()  [unwired: 5 in, 7 out]
        n411 = Insert Into Array(array=w854, index=0, new element=w852) -> (w853:T7[])
      }
      frame "Get/Release Control" {
        n412 = Unbundle By Name(w886) -> ("Login"=w884:bool)
        n413 = case shown="False" w884 {
          tunnel: [T28."Disabled" ("Disabled") T28."Enabled" ("Disabled")] -> w883
          frame False {
          }
          frame True {
          }
        }
        n414 = local write "Main Tab"(enum32{"Main", "Live Graph", "Configure"}."Main" ("Main Tab")) -> ()
        n415 = disable-structure shown="Disabled" {
          disable-tunnel: w883 -> [w887 _]
          frame Disabled {
            n416 = property on="pb.Stop Profile" class="Bool"("DisabledEnum"=w887) -> ()  [unwired: 2 in, 2 out]
          }
          frame Enabled {
          }
        }
        n417 = property on="Live Data Tab" class="TabCtl (strict)"("DisabledEnum"=w883) -> ()  [unwired: 2 in, 2 out]
        n418 = property on="Main Tab" class="TabCtl (strict)"("DisabledEnum"=w883) -> ()  [unwired: 2 in, 2 out]
        n419 = property on="Bank 1" class="Clust (strict)"("DisabledEnum"=w883) -> ()  [unwired: 2 in, 2 out]
        n420 = property on="Bank 2" class="Clust (strict)"("DisabledEnum"=w883) -> ()  [unwired: 2 in, 2 out]
        n421 = property on="Pump Timers Tab" class="TabCtl (strict)"("DisabledEnum"=w883) -> ()  [unwired: 2 in, 2 out]
      }
      frame "Init Data File" {
        w890 = FALSE ("Running?")
        n422 = Unbundle By Name(w908) -> ("LS DAS Config.CA Number"=w903:string, "LS DAS Config.Data File Name"=w904:string, "LS DAS Config.Serial Numbers"=w891:string[])
        n423 = Empty String/Path?(string/path=w904) -> (empty?=w902:bool)
        n424 = Empty String/Path?(string/path=w903) -> (empty?=w901:bool)
        n425 = call "Remove illegal file characters.vi"("Filename In"=w903) -> ("Filename Out"=w899:string)  [unwired: 10 in]
        n426 = call "Remove illegal file characters.vi"("Filename In"=w904) -> ("Filename Out"=w898:string)  [unwired: 10 in]
        n427 = Or(x=w902, y=w901) -> (x .or. y?=w900:bool)
        n428 = Build Path(base path=path "u:/CA Numbers", name or relative path=w899) -> (appended path=w905:path)
        n429 = case shown="False" w900 {
          tunnel: w905 -> [_ w921]
          tunnel: w898 -> [_ w920]
          tunnel: [path "" ("LS Data Filepath") w919] -> w892
          tunnel: [FALSE TRUE] -> w897
          tunnel: [T28."Disabled and Grayed Out" ("Disabled") T28."Enabled" ("Disabled")] -> w896
          frame True {
          }
          frame False {
            n430 = call <vilib>:"Check if File or Folder Exists.vi"("path"=w921) -> ("error out"=w914:errorcluster, "file or folder exists?"=w915:bool, "dup path"=w916:path)  [unwired: 8 in]
            n431 = case shown="False" w915 {
              tunnel: w916 -> [w925 w926]
              tunnel: w914 -> [w922 w927]
              tunnel: [w923 w927] -> _
              tunnel: [w924 w926] -> w913
              frame False {
                n432 = Create Folder(path (use dialog)=w925, error in=w922) -> (created path=w924:path, error out=w923:errorcluster)  [unwired: 1 in, 1 out]
              }
              frame True {
              }
            }
            n433 = Build Path(base path=w913, name or relative path=w920) -> (appended path=w919:path)
          }
        }
        n434 = property on="Profile based record" class="Bool (strict)"("Value"=w897, "DisabledEnum"=w896) -> ()  [unwired: 2 in, 2 out]
        n435 = local write "CA Number:"(w899) -> ()
        n436 = local write "Data File Name:"(w898) -> ()
        n437 = Bundle By Name(cluster=T26 {"Running?"=FALSE, "Record"=FALSE, "Data Filepath"=path "", "Serial Numbers"=[]} ("LS Cluster In"), "Running?"=w890, "Record"=w890, "Data Filepath"=w892, "Serial Numbers"=w891) -> (w894:T26)
        n438 = Bundle By Name(cluster=w908, "LS DAS Config.CA Number"=w899, "LS DAS Config.Data File Name"=w898, "LS Data Filepath"=w892) -> (w907:T23)
        n439 = call "LS DAS Global.vi"("Mode"=T25."Main Writes", "LS Cluster In"=w894) -> ()  [unwired: 7 in, 7 out]
      }
      frame "Save LS Data" {
        # "Opens"
        n440 = Unbundle By Name(w932) -> ("LS Data"=w930:T8)
        n441 = Unbundle By Name(w930) -> ("Opens"=w929:i32[])
        n442 = Array Size(array=w929) -> (size(s)=w928:i32)
        n443 = case shown="10" w928 {
          tunnel: w930 -> [_ w935]
          frame Default {
          }
          frame 10 {
            n444 = Write to Binary File(file (use dialog)=path "c:/Monitored Statistics" ("Path"), data=w935) -> (refnum out=w934:refnum<file>, error out=w933:errorcluster)  [unwired: 4 in, 1 out]
            n445 = Close File(refnum=w934, error in=w933) -> ()  [unwired: 2 out]
          }
        }
      }
      frame "Check Serial Numbers" {
        n446 = Unbundle By Name(w942) -> ("LS DAS Config.Serial Numbers"=w938:string[])
        n447 = for {
          tunnel: w938 -> [w944] mode=indexing
          tunnel: [w943] -> w937 mode=indexing
          n448 = call "Remove illegal file characters.vi"("Filename In"=w944) -> ("Filename Out"=w943:string)  [unwired: 10 in]
        }
        n449 = Array To Cluster(array=w937) -> (cluster=w939:T33)
        n450 = Bundle By Name(cluster=w942, "LS DAS Config.Serial Numbers"=w937) -> (w941:T23)
        n451 = local write "LS Serial Numbers"(w939) -> ()
      }
      frame "Main Tab" {
        # "Justin wants Start Test, Stop Test, and Data File Name always unlocked\n\nSo moved Data File Name to where it wouldn't sit on top of another\ncontrol on another page when I made it float like the stop button"
        n452 = Unbundle By Name(w948) -> ("Main Tab"=w947:enum32{"Main", "Live Graph", "Configure"})
        n453 = case shown="\"Main\"" w947 {
          tunnel: [T28."Enabled" ("Disabled") T28."Disabled" ("Disabled")] -> w946
          tunnel: [TRUE ("Visible") FALSE ("Visible")] -> w945
          frame "Main" {
          }
          frame Default {
          }
        }
        n454 = property on="pb.Run Profile" class="Bool (strict)"("Visible"=w945, "DisabledEnum"=w946) -> ()  [unwired: 2 in, 2 out]
        n455 = property on="Data File Name:" class="Str"("Visible"=w945, "DisabledEnum"=w946) -> ()  [unwired: 2 in, 2 out]
      }
      frame "Allow Data Note" {
        w958 = T7[] [enum."Enable Background"] items=["Main", "Init Files", "Init", "Unused", "Save As", "Start Profile", "Check Step Time", "Alarm", "Alarm Dismiss", "Run Step", "Stop Profile", "Cycle Reset", "Time Reset", "Time Reset All", "Time Set", "Tare CTs", "Save Profile", "Open Profile", "Get Profiles", "Update Screen", "Update Controls", "Save App Config", "Write Outputs", "Disable Background", "Enable Background", "Get/Release Control", "Log Fuel Change", "Fuel Change Popup", "Read Inputs", "Remote Timer Reset", "Controller Change", "Get Alarms", "Init Alarms", "Save Alarms", "Voltage Selection", "Set Watlow Temp 1", "Set Watlow Temp 2", "Get Pressure", "Write Tare Pressure", "Adjust Controls", "Reinit ADC", "Write Initial Times", "Write Pumps Present", "HMI Command", "Save Pump Times", "Check Pump Stop Time", "Save LS App Config", "Init Data File", "Reset LS Cycles", "Reset Anomalies", "Reset Opens", "Save LS Data", "Save LS Test Data", "Check Serial Numbers", "Main Tab", "Allow Data Note", "Resume Profile", "Pause Profile", "Allow Pause Note", "Clear Graph"]
        n456 = flat-sequence {
          tunnel: [w967] -> w956
          tunnel: w957 -> [w966]
          tunnel: [w965] -> w955
          tunnel: w956 -> [w979]
          tunnel: w955 -> [w978]
          tunnel: [w975] -> w954
          tunnel: w954 -> [w988]
          frame #0 {
            w962 = FALSE ("Visible")
            n457 = property on="Cycle Pts to Avg:" class="DigNum (strict)"("Visible"=w962) -> ()  [unwired: 2 in, 2 out]
            n458 = property on="Cycle Threshold:" class="DigNum (strict)"("Visible"=w962) -> ()  [unwired: 2 in, 2 out]
            n459 = property on="pb.Stop Profile" class="Bool"("Visible"=w962) -> ()  [unwired: 2 in, 2 out]
            n460 = property on="Data File Name:" class="Str"("Visible"=w962) -> ()  [unwired: 2 in, 2 out]
            n461 = property on="pb.Run Profile" class="Bool (strict)"("Visible"=w962) -> ()  [unwired: 2 in, 2 out]
            n462 = property on="Bank 1 Voltage Offset:" class="DigNum (strict)"("Visible"=w962) -> ()  [unwired: 2 in, 2 out]
            n463 = property on="Bank 2 Voltage Offset:" class="DigNum (strict)"("Visible"=w962) -> ()  [unwired: 2 in, 2 out]
            n464 = property on="Note Tab" class="TabCtl (strict)"("Visible"=TRUE) -> ()  [unwired: 2 in, 2 out]
            n465 = property on="Main Tab" class="TabCtl (strict)"("DisabledEnum"=T28."Enabled" ("Disabled")) -> ()  [unwired: 2 in, 2 out]
          }
          frame #1 {
            n466 = while {
              tunnel: ["pb.Note OK"] -> w969
              stop <- w973 stop-if-true
              n467 = Wait (ms)(milliseconds to wait=u32 10) -> ()  [unwired: 1 out]
              n468 = local write "Main Tab"(enum32{"Main", "Live Graph", "Configure"}."Configure" ("Main Tab")) -> ()
              n469 = Or(x="pb.Note Cancel", y="pb.Note OK") -> (x .or. y?=w973:bool)
            }
            n470 = Unbundle By Name(w966) -> ("Login"=w965:bool, "LS DAS Config.Profile Record"=w968:bool)
            n471 = And(x=w968, y=w969) -> (x .and. y?=w967:bool)
          }
          frame #2 {
            n472 = case shown="True" w979 {
              frame False {
              }
              frame True {
                w983 = "\n"
                n473 = Concatenate Strings("Stop, Button, Pressed", w983, "Note:,", "Stop Profile Note", w983) -> (w981:string)
                n474 = call "LS DAS Global.vi"("Mode"=T25."Write Note", "Note IN"=w981) -> ()  [unwired: 7 in, 7 out]
              }
            }
            n475 = Select(t=T28."Enabled" ("Disabled"), s=w978, f=T28."Disabled" ("Disabled")) -> (s? t:f=w975:T28)
          }
          frame #3 {
            w986 = TRUE ("Visible")
            n476 = local write "Stop Profile Note"("" ("Stop Profile Note")) -> ()
            n477 = property on="Cycle Pts to Avg:" class="DigNum (strict)"("Visible"=w986) -> ()  [unwired: 2 in, 2 out]
            n478 = property on="Cycle Threshold:" class="DigNum (strict)"("Visible"=w986) -> ()  [unwired: 2 in, 2 out]
            n479 = property on="pb.Stop Profile" class="Bool"("Visible"=w986) -> ()  [unwired: 2 in, 2 out]
            n480 = property on="Data File Name:" class="Str"("Visible"=w986) -> ()  [unwired: 2 in, 2 out]
            n481 = property on="pb.Run Profile" class="Bool (strict)"("Visible"=w986) -> ()  [unwired: 2 in, 2 out]
            n482 = property on="Bank 1 Voltage Offset:" class="DigNum (strict)"("Visible"=w986) -> ()  [unwired: 2 in, 2 out]
            n483 = property on="Bank 2 Voltage Offset:" class="DigNum (strict)"("Visible"=w986) -> ()  [unwired: 2 in, 2 out]
            n484 = local write "Main Tab"(enum32{"Main", "Live Graph", "Configure"}."Main" ("Main Tab")) -> ()
            n485 = property on="Main Tab" class="TabCtl (strict)"("DisabledEnum"=w988) -> ()  [unwired: 2 in, 2 out]
            n486 = property on="Note Tab" class="TabCtl (strict)"("Visible"=FALSE) -> ()  [unwired: 2 in, 2 out]
          }
        }
        n487 = Insert Into Array(array=w961, index=0, new element=w958) -> (w960:T7[])
      }
      frame "Clear Graph" {
        n488 = property on="Waveform Chart" class="WFChart (strict)"("History Data"=dbl[] []) -> ()  [unwired: 2 in, 2 out]
      }
    }
  }
  n489 = flat-sequence {
    tunnel: w10 -> [_]
    tunnel: w9 -> [w994]
    frame #0 {
      n490 = call "LS DAS Loop.vi"("FPGA Ref"=w994) -> ()  [unwired: 11 in]
      n491 = disable-structure shown="Disabled" {
        frame Disabled {
          n492 = call "Email Loop.vi"() -> ()  [unwired: 12 in]
        }
        frame Enabled {
        }
      }
      n493 = call "App Loop.vi"() -> ()  [unwired: 12 in]
    }
  }
  n494 = while {
    tunnel: w9 -> [w997]
    stop <- FALSE stop-if-true
    n495 = local read "Main Tab"() -> (w995:enum32{"Main", "Live Graph", "Configure"})
    n496 = case shown="\"Live Graph\"" w995 {
      tunnel: w997 -> [_ w1000]
      frame Default {
        n497 = Wait (ms)(milliseconds to wait=u32 10) -> ()  [unwired: 1 out]
      }
      frame "Live Graph" {
        n498 = case shown="False" "Pause" {
          tunnel: w1000 -> [w1005 _]
          frame False {
            n499 = xnode "Read/Write Control"("FPGA VI Reference In"=w1005) -> ("Anomaly Resamples"=w1003:fxp<+/-,28,17>[])  [unwired: 1 in, 2 out]
            n500 = Index Array(array=w1003, index="Graph Selection") -> (element=→"Waveform Chart":fxp<+/-,28,17>)
            n501 = Wait (ms)(milliseconds to wait=u32 1) -> ()  [unwired: 1 out]
          }
          frame True {
            n502 = Wait (ms)(milliseconds to wait=u32 10) -> ()  [unwired: 1 out]
          }
        }
      }
    }
  }
